vi "Preference_Panel.vi"(0 "Mode":T3) -> ()   [LabVIEW 2015]
uses:
  Anemometry Sub Vis/Controls/Server_Comms.ctl
  Anemometry Sub Vis/Controls/Preference_Mode.ctl
  Anemometry Sub Vis/Controls/EnFlo_Data_Folder_Setup.ctl
  Camera Server/Camera enum/Camera enum.ctl
  Anemometry Sub Vis/File/Setup_Filetype.ctl
  Anemometry Sub Vis/Controls/Overhead.ctl
  ADAM Client/Sub VIs/ADAM Controls/Ch_description_ADAM.ctl
  ADAM Client/Sub VIs/ADAM Controls/Module_type_ADAM.ctl
  ADAM Client/Sub VIs/ADAM Controls/Function_ADAM.ctl
  ADAM Client/Sub VIs/ADAM Controls/Channel_State.ctl
  ADAM Client/Sub VIs/ADAM Controls/Calib_type_ADAM.ctl
  ADAM Client/Sub VIs/ADAM Controls/Address.ctl
  Anemometry Sub Vis/Globals/Constants_global.vi
  Anemometry Sub Vis/Globals/Preference_global.vi
  Anemometry Sub Vis/Globals/Trav_pos_global.vi
  Camera Server/Globals/CamServer global.vi
  Anemometry Sub Vis/Acquisition/PWA/PWAtasksGLOBAL.vi
panel:
  in  "Cameras to Log":T1[](array[typedef])
  out "Preferences for computer":string
  in  "Log Cameras if available":bool
  in  "Use New Collision Code":bool
  in  "Traverse to Traverse Collision Detection":bool
  in  "DataTranslation Device No.":u32=20
  in  "Reset Email Counter":bool
  in  "EnFlo_Data_Folder_Setup":T2="EnFlo_Data on Server"
  in  "Post Processing Machine":bool
  in  "Analogue Device Serial No.":string="1188AB4"
  in  "PWA Device Serial No.":string="1187C98"
  in  "ADAM Setup File":u16(ring) items=["Current_Setup.xls"]
  in  "Default Source Establishment Time (s)":dbl=20.0
  out "This Machine's IP Number":string
  in  "Rig Setup":u16(ring) items=["3_x_2_tunnel", "A_Tunnel", "ADAM_Server", "Aero_Server", "Aero_Tunnel", "B_Tunnel", "Bench_Blower", "Contact_Conductance", "D_Tunnel", "EES_Project", "EnFlo_Tunnel", "Fruit_Rig", "Jet_Engine", "Laser_Disp_Scanner", "Paul_Hayden_Desk", "Post_Processing_Machine", "Soil_Rig", "Synthetic_Jet", "Tank", "TF_Standalone", "Wind_Turbine_Blade_Setup", "--New Rig Setup--"]
  in  "Default Traverse Name":u16(ring) items=["A_Tunnel", "Aero_Enclosure", "Aero_Sting", "Aero_ThroughWall", "Aero_Tunnel", "Angle_Calibrator", "B_Tunnel", "D_Tunnel", "dummy", "Dummy_Traverse", "EnFlo_", "EnFlo_Measure_Height", "EnFlo_Stack", "EnFlo_Stack  dfg", "EnFlo_Trav3", "EnFlo_Tunnel", "EnFlo_Turntable", "Fruit_Rig", "Hello_5.xls", "Laser_Disp_Scanner", "Laser_Meas_Traverse", "None", "Pitch_Traverse", "Pitch_Yaw", "PIV_Traverse", "Pressure_Port_1", "Pressure_Port_2", "Scanning Valve", "Soil_Rig", "Tank", "--New Traverse Setup--"]
  in  "OK":bool
  in  "% Error From First Calib":dbl=10.0 format="%.1f"
  in  "% Error From Previous Calib":dbl=0.5 format="%.1f"
  out "Templates":path=path "/G4_2_HD/Applications (Mac OS 9)/EnFlo Software/Anemometry/Anemometry Sub Vis/Templates"
  in  "Data Folder":path
  out "EnFlo SW Preferences":path=path "/G4_2_HD/Applications (Mac OS 9)/LabVIEW 5.1/EnFlo SW Preferences"
  in  "Tunnel Speed Control":bool
  in  "SMTP server IP address":string
  in  "Abs Press (mbar)":string="Froude:NPL:Atmos_Press"
  in  "Temperature":string="EnFlo Tun:Inlet Heater:Av Temp"
  in  "Server port number":u32=3363
  in  "Server address":string
  in  "LabVIEW Administrators":string[](array[string])=["", "", "", "", "", "", "", "", "", "", "", "", "", "", "", "", "", "", "", ""]
  in  "Server Comms":T4=enum."Do Not Link To Server"
  # "Server Computer Peferences"
  # "Multi Run Preferences"
  # "Warning Levels for Autocalibration Changes"
  # "Email Peferences"
  # "Deg C"
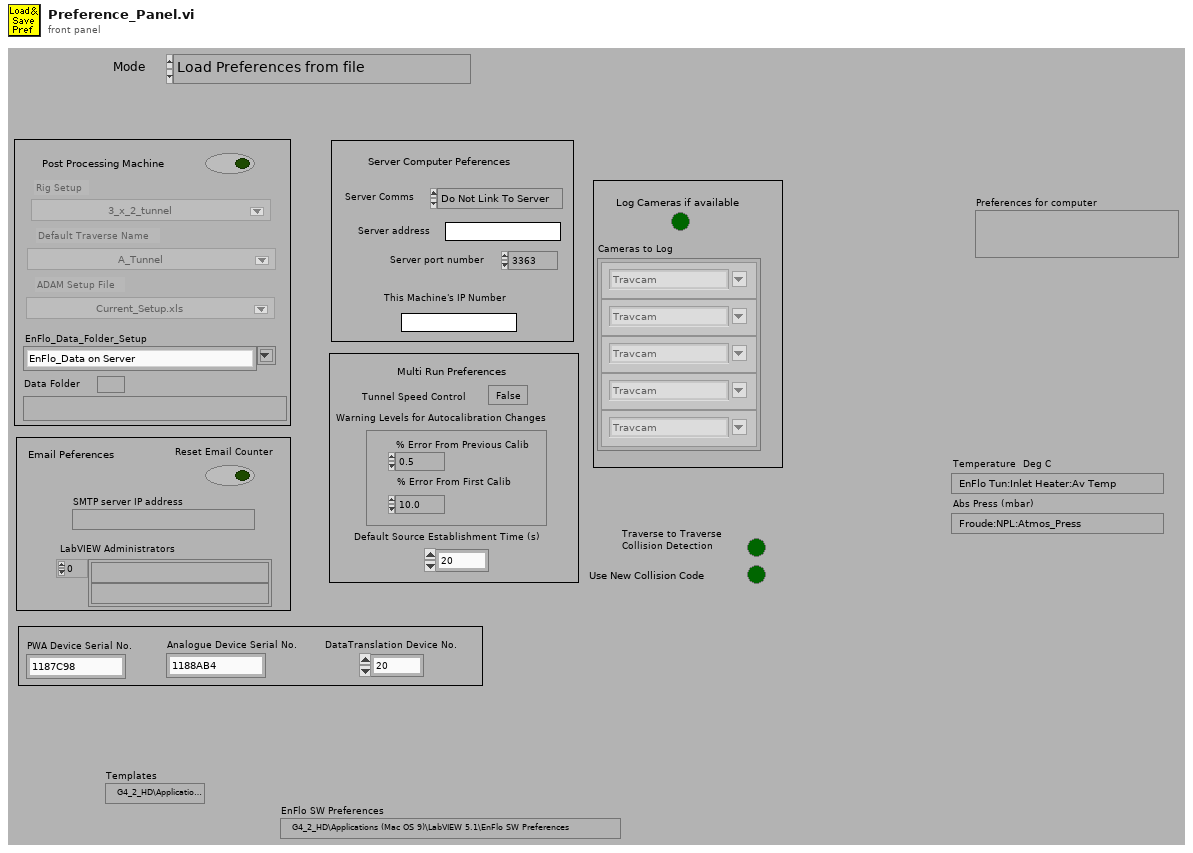
[diagram p1: front panel]
types:
  T1 = typedef "Camera enum.ctl" = string
  T2 = typedef "EnFlo_Data_Folder_Setup.ctl" = string
  T3 = typedef "Preference_Mode.ctl" = enum16{"Load Preferences from file", "Save Preferences to file", "Load, Edit then Save"}
  T4 = typedef "Server_Comms.ctl" = enum16{"Server Link Healthy", "Do Not Link To Server"}
  T5 = enum16{"Zero or one", "One", "Zero or more", "One or more"}
  T6 = enum8{"Enabled", "Disabled", "Disabled and Grayed Out"}
  T7 = typedef "Setup_Filetype.ctl" = enum16{"Measurement Setups", "Calibration Setups", "General", "Results File Plotter Setups", "Speed Calib Tweaks"}
  T8 = typedef "Overhead.ctl" = enum16{"Update total times", "Read Current Overhead", "Re Scale totals to 3 hrs", "Initialise totals to 3hr"}
  T9 = typedef "Calib_type_ADAM.ctl" = enum16{"Raw", "Bx + A", "Cx^2 + Bx + A", "Dx^3 + Cx^2 + Bx + A", "In Band", "Hi-Tec Q", "Hi-Tec M_dot", "Text"}
  T10 = typedef "Module_type_ADAM.ctl" = string
  T11 = typedef "Channel_State.ctl" = enum16{"On", "Off", "Always On", "Always Off"}
  T12 = typedef "LVDateTimeRec.ctl" = cluster{"fractional second":dbl, "second":i32, "minute":i32, "hour":i32, "day of month":i32, "month":i32, "year":i32, "day of week":i32, "day of year":i32, "DST":i32}
  T13 = typedef "Ch_description_ADAM.ctl" = cluster{"Ch Name":string, "Type":T10, "Function":T14, "Ch State":T11, "Calibration type":T9, "A":dbl, "B":dbl, "C":dbl, "D":dbl, "Comments":string, "Address":T15, "String":string, "Duty":u16}
  T14 = typedef "Function_ADAM.ctl" = enum16{"Analogue Input", "Digital Input", "Event counter", "Event rate", "Analogue Output", "Digital Output", "Relay Output"}
  T15 = typedef "Address.ctl" = cluster{"Main":i32, "Ch.":i32, "Sub":i32, "Port Name":string}
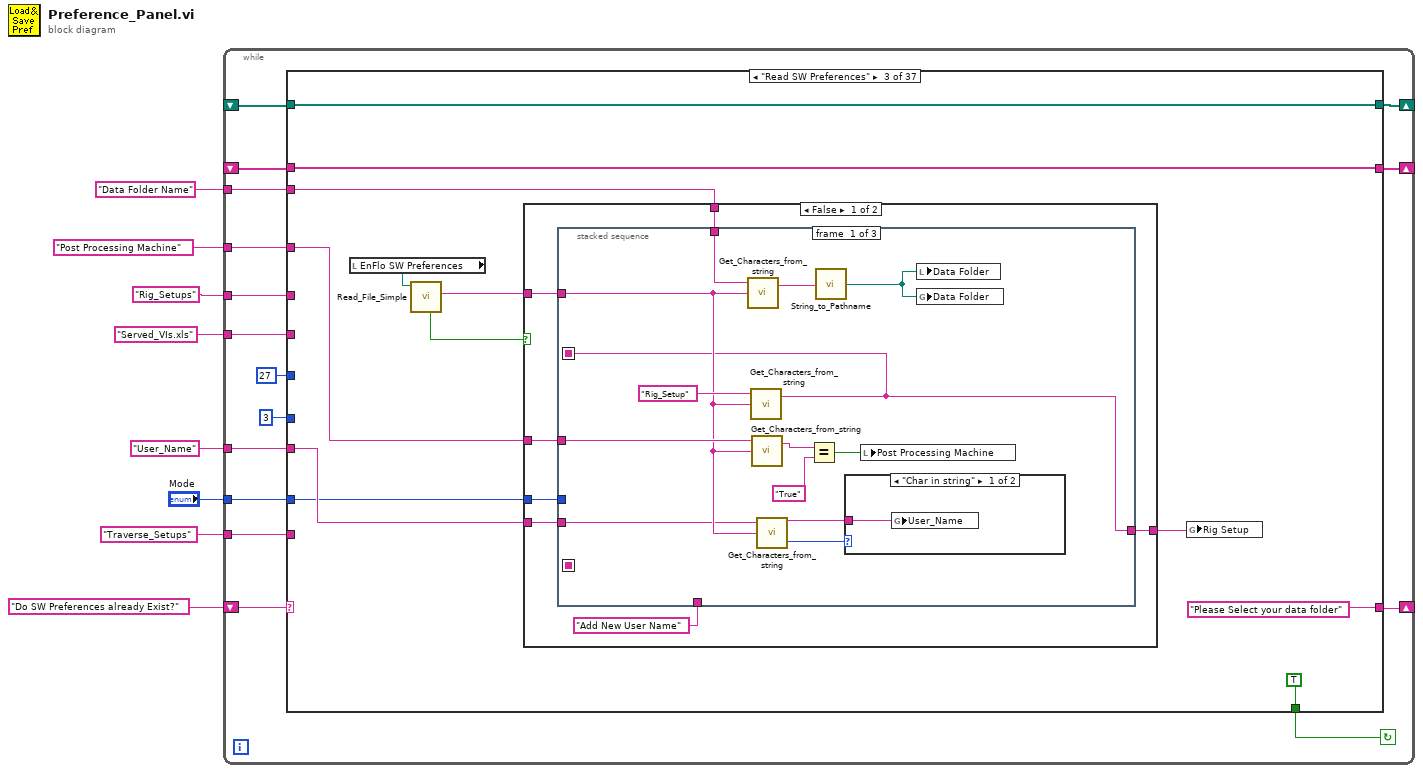
[diagram p0: block diagram]
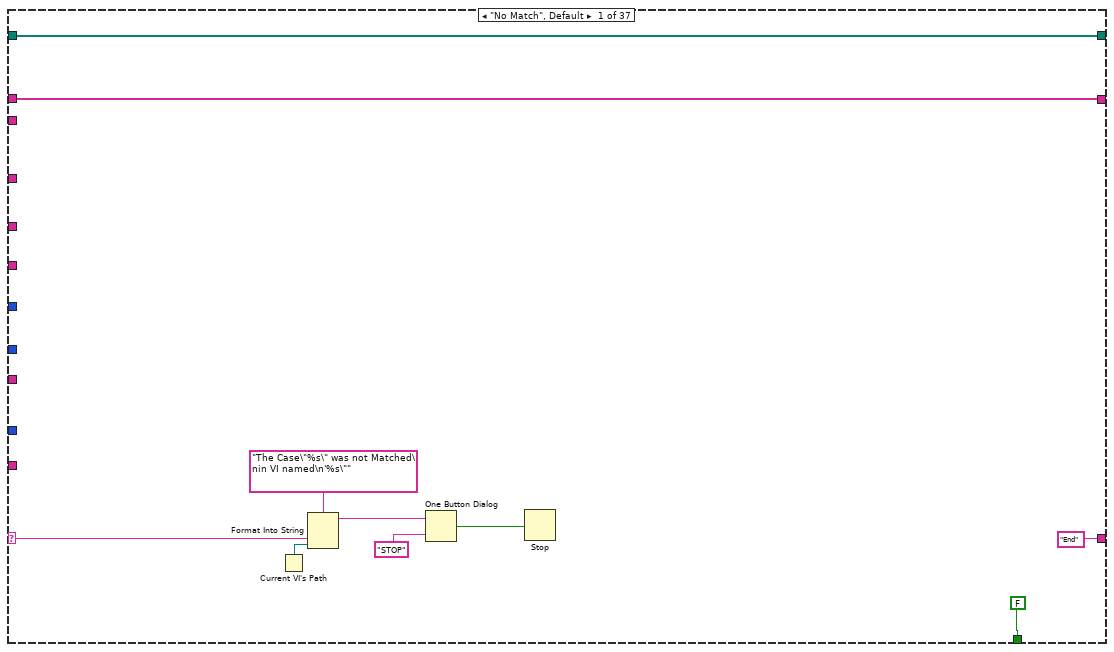
[diagram p2: hidden frame]
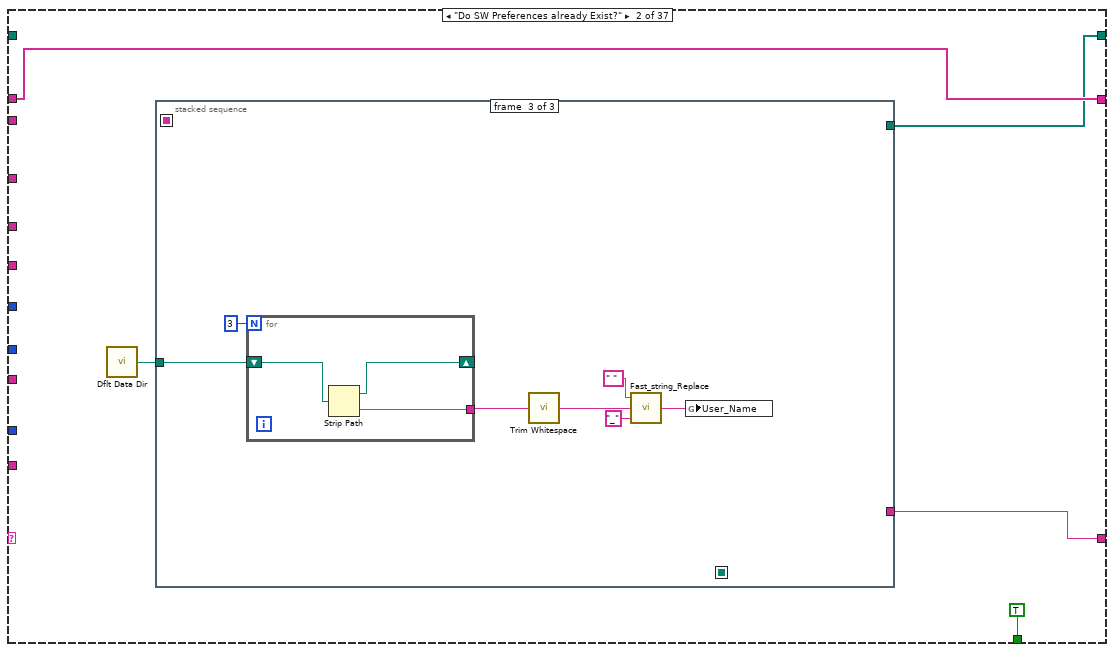
[diagram p3: hidden frame]
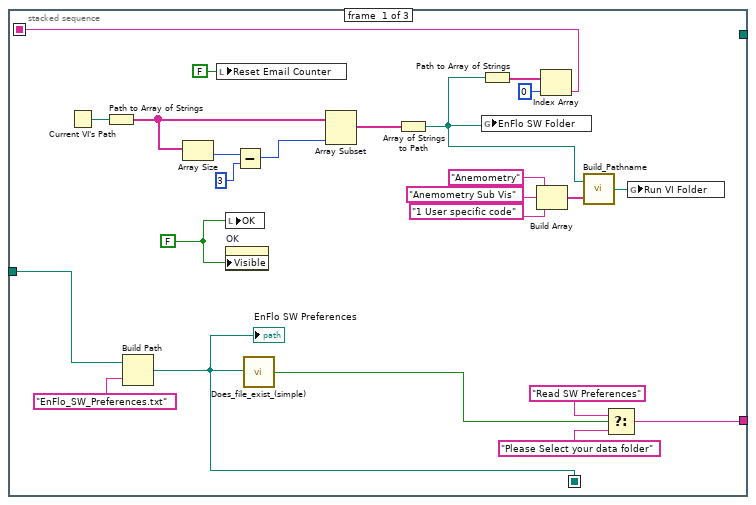
[diagram p4: hidden frame]
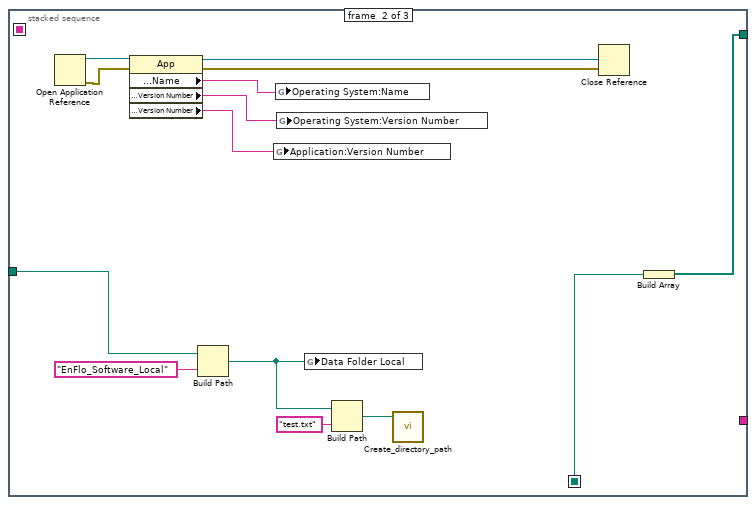
[diagram p5: hidden frame]
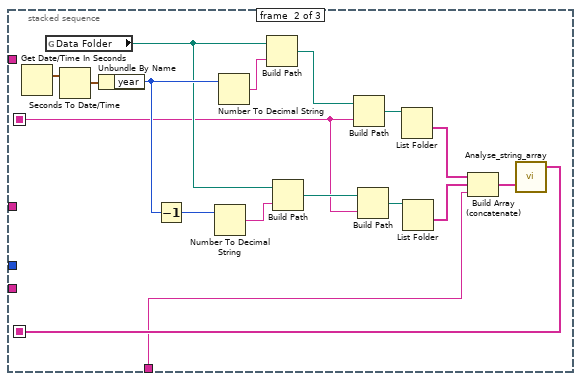
[diagram p7: hidden frame]
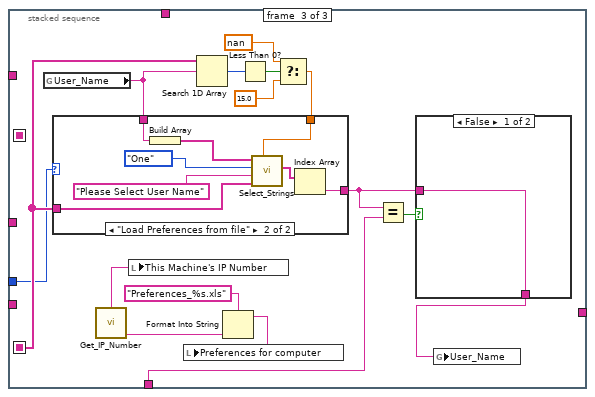
[diagram p8: hidden frame]
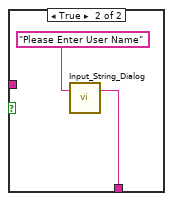
[diagram p10: hidden frame]
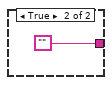
[diagram p11: hidden frame]
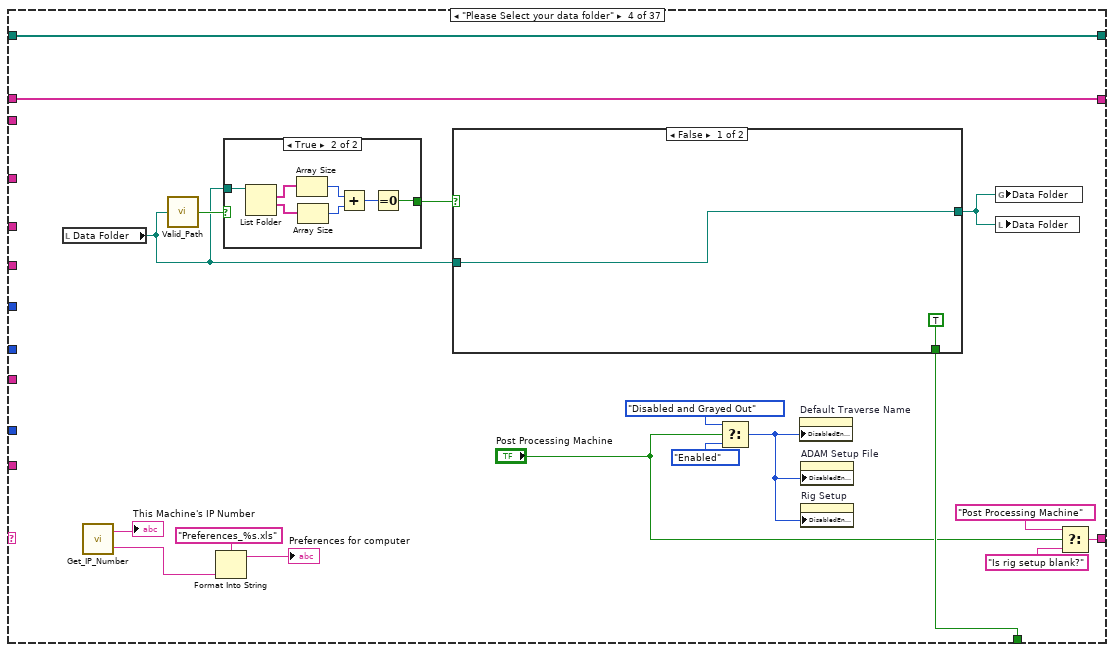
[diagram p12: hidden frame]
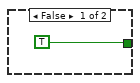
[diagram p13: hidden frame]
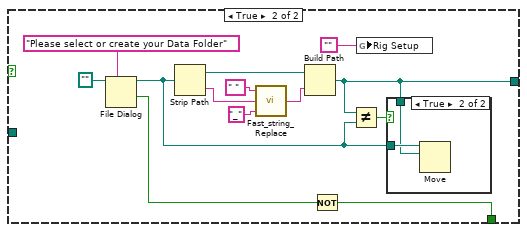
[diagram p14: hidden frame]
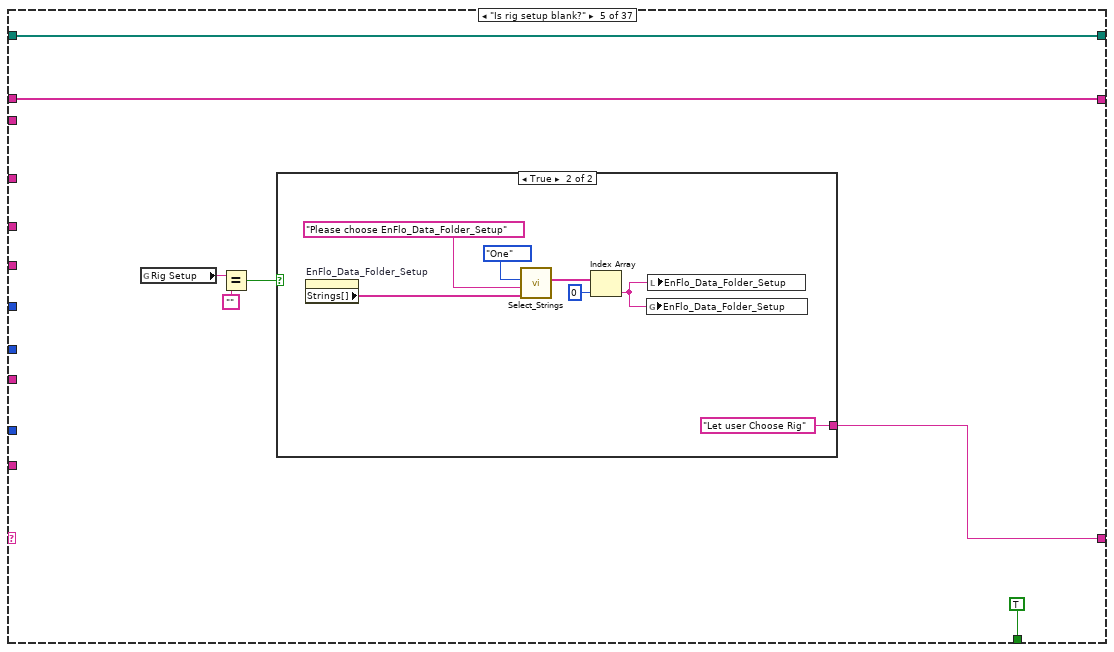
[diagram p16: hidden frame]
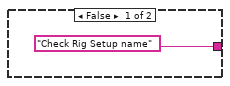
[diagram p17: hidden frame]
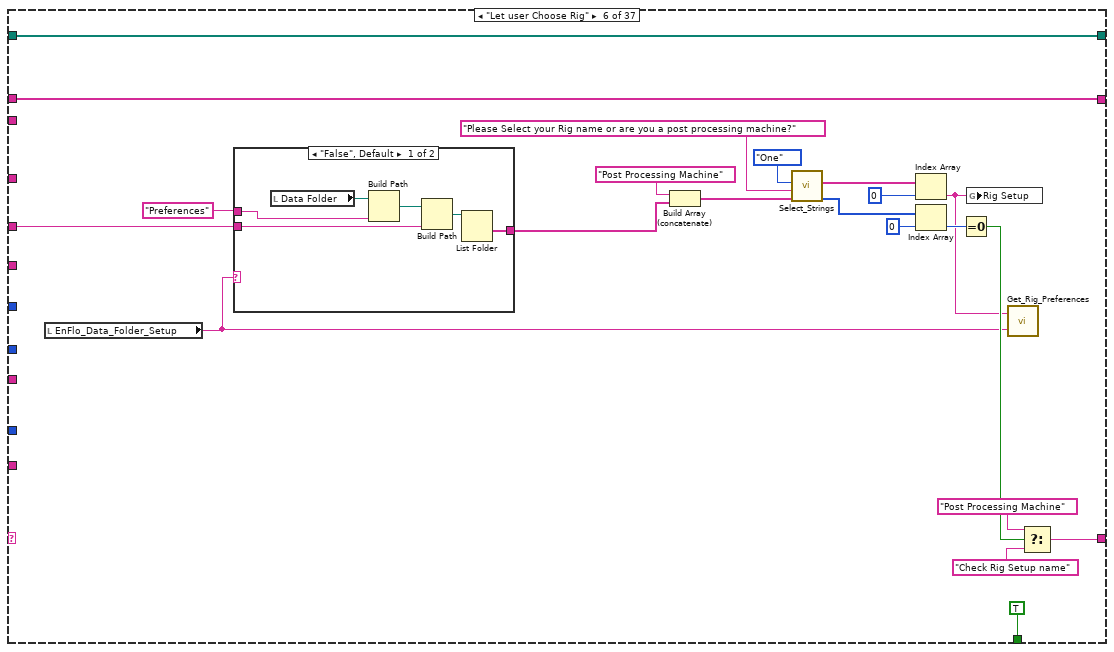
[diagram p18: hidden frame]
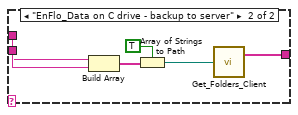
[diagram p19: hidden frame]
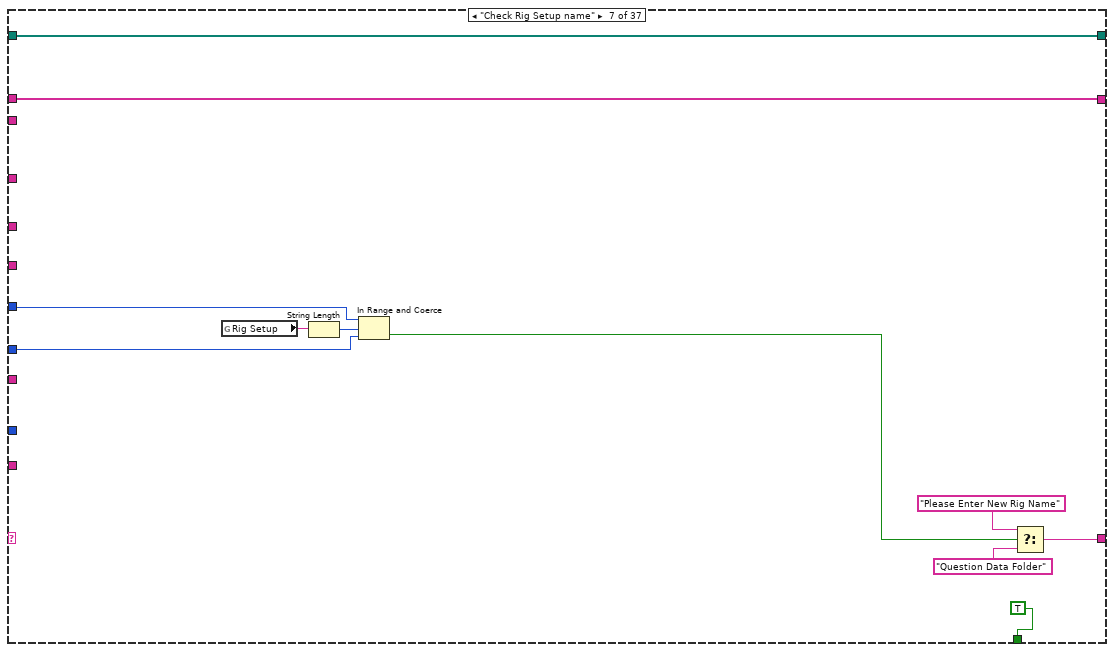
[diagram p20: hidden frame]
diagram:
  n1 = while {
    shift-left: _ -> [w21]
    shift-right: [w22] -> _
    shift-left: "Do SW Preferences already Exist?" -> [w10]
    shift-right: [w23] -> _
    tunnel: "Mode" -> [w20]
    tunnel: "Data Folder Name" ("Label for characters") -> [w19]
    tunnel: "Served_VIs.xls" ("Substring") -> [w18]
    tunnel: "Rig_Setups" ("Folder") -> [w15]
    tunnel: "Traverse_Setups" ("name or relative path") -> [w14]
    shift-right: [w13] -> _
    shift-left: _ -> [w12]
    tunnel: "Post Processing Machine" ("Label for characters") -> [w11]
    tunnel: "User_Name" ("Label for characters") -> [w9]
    stop <- w24 continue-if-true
    n2 = case shown="\"Read SW Preferences\"" w10 {
      selector: w10 -> [w25 _ _ _ _ _ _ _ _ _ _ _ _ _ _ _ _ _ _ _ _ _ _ _ _ _ _ _ _ _ _ _ _ _ _ _ _]
      tunnel: [FALSE TRUE TRUE w178 TRUE TRUE TRUE TRUE TRUE TRUE TRUE TRUE TRUE TRUE TRUE TRUE TRUE TRUE TRUE TRUE TRUE TRUE TRUE TRUE TRUE TRUE TRUE TRUE TRUE TRUE TRUE TRUE w940 TRUE TRUE TRUE FALSE] -> w24
      tunnel: ["End" w37 "Please Select your data folder" w175 w210 w241 w258 w269 w288 "Update Constants Global" ("f") "Copy Preferences?" "Copy Preferences?" w419 w436 "Install Preference files" "Install Adam table files" "Install Adam setup files" "Choose ADAM Setup file" "Preference files continued" "Variable Names" w613 w633 "Please Enter new  Traverse Setup" w720 "Create Traverse setup" ("f") "Check file permission status" w817 w848 w868 w888 w904 "Save Preference File" "Save SW Preferences" w1030 w1044 "Initialise Globals" "End"] -> w23
      tunnel: [w27 w38 w98 w184 w215 w244 w267 w277 w290 w355 w383 w406 w417 w439 w495 w510 w535 w554 w576 w586 w618 w640 w708 w722 w756 w773 w818 w853 w873 w896 w909 w929 w946 w1038 w1045 w1097 w1155] -> w22
      tunnel: w21 -> [w27 w38 w98 w184 w215 w244 w267 w277 w290 w355 w383 w406 w417 w439 w495 w510 w535 w554 w576 w586 _ w640 w708 w722 w756 w773 w818 w853 w873 w896 w909 w929 w946 w1038 w1045 w1097 w1155]
      tunnel: w20 -> [_ _ w88 _ _ _ _ _ _ _ _ _ _ _ _ _ _ _ _ _ w612 _ _ _ _ _ w816 _ _ _ _ _ w941 _ _ _ _]
      tunnel: w19 -> [_ _ w95 _ _ _ _ _ _ _ _ _ _ _ _ _ _ _ _ _ _ _ _ _ _ _ _ _ _ _ _ _ _ w1029 _ _ _]
      tunnel: w18 -> [_ _ _ _ _ _ _ _ _ _ _ _ _ _ _ w505 _ _ _ _ _ _ _ _ _ _ _ _ _ _ _ _ _ _ _ w1089 _]
      tunnel: 3 ("lower limit") -> [_ _ _ _ _ _ w263 _ w287 _ _ _ _ _ _ _ _ _ _ _ _ _ _ w719 _ _ _ _ _ _ _ _ _ _ _ _ _]
      tunnel: 27 ("upper limit") -> [_ _ _ _ _ _ w264 _ w286 _ _ _ _ _ _ _ _ _ _ _ _ _ _ w718 _ _ _ _ _ _ _ _ _ _ _ _ _]
      tunnel: w15 -> [_ _ _ _ _ w229 _ _ _ w343 w372 _ _ _ _ _ _ _ _ _ _ _ _ _ _ _ _ _ _ _ _ _ _ _ _ _ _]
      tunnel: w14 -> [_ _ _ _ _ _ _ _ _ _ _ _ _ _ _ _ _ _ _ _ _ _ w706 _ w743 _ _ _ _ _ _ _ _ _ _ _ _]
      tunnel: [w26 w35 w94 w179 w211 w243 w266 w276 w282 w341 w369 w396 w418 w440 w488 w502 w528 w551 w562 w578 w605 w636 w705 w714 w742 w769 path[] [] w845 w865 w891 w907 w928 w939 w1026 w1043 w1091 w1153] -> w13
      tunnel: w12 -> [w26 _ w94 w179 w211 w243 w266 w276 w282 w341 w369 w396 w418 w440 w487 w504 w528 w552 w562 w580 w605 w637 w705 w714 w742 w770 w815 w845 w865 w891 w907 w928 w939 w1026 w1043 w1091 w1153]
      tunnel: w11 -> [_ _ w93 _ _ _ _ _ _ _ _ _ _ _ _ _ _ _ _ _ _ _ _ _ _ _ _ _ _ _ _ _ _ w1020 _ _ _]
      tunnel: w9 -> [_ _ w89 _ _ _ _ _ _ _ _ _ _ _ _ _ _ _ _ _ _ _ _ _ _ _ _ _ _ _ _ _ _ w1019 _ _ _]
      frame "No Match", Default {
        n3 = Current VI's Path() -> (path=w34:path)
        n4 = Format Into String(format string="The Case\"%s\" was not Matched\nin VI named\n'%s\"" ("Format String"), w25, w34) -> (resulting string=w31:string)  [unwired: 2 in, 1 out]
        n5 = One Button Dialog(message=w31, button name ("OK")="STOP") -> (true=w33:bool)
        n6 = Stop(stop? (T)=w33) -> ()
      }
      frame "Do SW Preferences already Exist?" {
        n7 = call <vilib>:"Dflt Data Dir.vi"() -> ("App:Default Data Directory"=w36:path)
        n8 = stacked-sequence {
          seq-local: [w50 _ _] -> [_ _ _]
          seq-local: [w48 _ _] -> [_ w69 _]
          tunnel: [w53 _ _] -> w37
          tunnel: w36 -> [w49 w67 w83]
          tunnel: [_ w70 _] -> w35
          frame #0 {
            w47 = FALSE ("OK")
            n9 = Current VI's Path() -> (path=w61:path)
            n10 = Path to Array of Strings(0:w61) -> (2:w58:string[])  [unwired: 1 out]
            n11 = Build Path(base path=w49, name or relative path="EnFlo_SW_Preferences.txt") -> (appended path=w48:path)
            "EnFlo SW Preferences" <- w48
            n12 = Array Size(array=w58) -> (size(s)=w60:i32)
            n13 = local write "Reset Email Counter"(FALSE ("Reset Email Counter")) -> ()
            n14 = local write "OK"(w47) -> ()
            n15 = property on="OK" class="Bool (strict)"("Visible"=w47) -> ()  [unwired: 2 in, 2 out]
            n16 = Subtract(x=w60, y=3) -> (x-y=w56:i32)
            n17 = call "Does_file_exist_(simple).vi"("Pathname"=w48) -> ("exists?"=w62:bool)
            n18 = Array Subset(array=w58, length=w56) -> (w57:string[])  [unwired: 1 in]
            n19 = Array of Strings to Path(0:w57) -> (2:w45:path)  [unwired: 1 out]
            n20 = Path to Array of Strings(0:w45) -> (2:w51:string[])  [unwired: 1 out]
            n21 = global write "Constants_global.vi" "EnFlo SW Folder"(w45) -> ()
            n22 = Build Array("Anemometry" ("name or relative path"), "Anemometry Sub Vis" ("name or relative path"), "1 User specific code" ("name or relative path")) -> (w40:string[])
            n23 = Index Array(array=w51, index=0) -> (element=w50:string)
            n24 = call "Build_Pathname.vi"("PathElements"=w40, "PathnameIn"=w45) -> ("AppendedPath"=w44:path)
            n25 = Select(t="Read SW Preferences", s=w62, f="Please Select your data folder") -> (s? t:f=w53:string)
            n26 = global write "Constants_global.vi" "Run VI Folder"(w44) -> ()
          }
          frame #1 {
            n27 = Open Application Reference() -> (0:w74:errorcluster, 3:w77:refnum<vi>)  [unwired: 1 in, 3 out]
            n28 = property class="App"(reference=w77, error in=w74) -> (reference out=w76:refnum<vi>, error out=w75:errorcluster, "Operating System:Name"=w71:string, "Operating System:Version Number"=w73:string, "Application:Version Number"=w72:string)
            n29 = Build Path(base path=w67, name or relative path="EnFlo_Software_Local" ("element")) -> (appended path=w66:path)
            n30 = global write "Preference_global.vi" "Application:Version Number"(w72) -> ()
            n31 = global write "Preference_global.vi" "Operating System:Name"(w71) -> ()
            n32 = global write "Preference_global.vi" "Operating System:Version Number"(w73) -> ()
            n33 = global write "Constants_global.vi" "Data Folder Local"(w66) -> ()
            n34 = Build Path(base path=w66, name or relative path="test.txt") -> (appended path=w64:path)
            n35 = call "Create_directory_path.vi"("Path name"=w64) -> ()  [unwired: 2 in, 2 out]
            n36 = Close Reference(reference=w76, error in (no error)=w75) -> ()  [unwired: 1 out]
            n37 = Build Array(w69) -> (w70:path[])
          }
          frame #2 {
            n38 = for {
              N: 3 -> [_]
              shift-right: [w87] -> _
              shift-left: w83 -> [w86]
              tunnel: [w85] -> w79
              n39 = Strip Path(path=w86) -> (stripped path=w87:path, name=w85:string)
            }
            n40 = call <vilib>:"Trim Whitespace.vi"("string"=w79) -> ("trimmed string"=w78:string)  [unwired: 1 in]
            n41 = call "Fast_string_Replace.vi"("Replace match with:"="_", "Input String"=w78, "regular expression"=" ") -> ("Output String"=w80:string)  [unwired: 1 in, 1 out]
            n42 = global write "Preference_global.vi" "User_Name"(w80) -> ()
          }
        }
      }
      frame "Read SW Preferences" {
        n43 = local read "EnFlo SW Preferences"() -> (w97:path)
        n44 = call "Read_File_Simple.vi"("Filename"=w97) -> ("Error?"=w91:bool, "string"=w92:string)  [unwired: 2 in, 6 out]
        n45 = case shown="False" w91 {
          tunnel: w95 -> [w106 _]
          tunnel: w93 -> [w105 _]
          tunnel: w92 -> [w103 _]
          tunnel: [w104 ""] -> w90
          tunnel: w89 -> [w102 _]
          tunnel: w88 -> [w100 _]
          frame False {
            n46 = stacked-sequence {
              seq-local: [w109 _ _] -> [_ w127 _]
              seq-local: [_ w122 _] -> [_ _ w148]
              tunnel: w106 -> [w119 _ _]
              tunnel: w105 -> [w117 _ _]
              tunnel: [w109 _ _] -> w104
              tunnel: w103 -> [w113 _ _]
              tunnel: w102 -> [w112 _ _]
              tunnel: "Add New User Name" -> [_ w121 w153]
              tunnel: w100 -> [_ _ w138]
              frame #0 {
                n47 = call "Get_Characters_from_string.vi"("Input string"=w113, "Variable name"=w119) -> ("Value"=w108:string)  [unwired: 1 in, 1 out]
                n48 = call "Get_Characters_from_string.vi"("Input string"=w113, "Variable name"="Rig_Setup" ("Label for characters")) -> ("Value"=w109:string)  [unwired: 1 in, 1 out]
                n49 = call "Get_Characters_from_string.vi"("Input string"=w113, "Variable name"=w117) -> ("Value"=w116:string)  [unwired: 1 in, 1 out]
                n50 = call "Get_Characters_from_string.vi"("Input string"=w113, "Variable name"=w112) -> ("Status"=w111:enum16{"Char in string", "Char not in string"}, "Value"=w110:string)  [unwired: 1 in]
                n51 = Equal?(x=w116, y="True") -> (x = y?=w114:bool)
                n52 = call "String_to_Pathname.vi"("Input String"=w108) -> ("path"=w107:path)
                n53 = case shown="\"Char in string\"" w111 {
                  tunnel: w110 -> [w120 _]
                  frame "Char in string" {
                    n54 = global write "Preference_global.vi" "User_Name"(w120) -> ()
                  }
                  frame "Char not in string" {
                  }
                }
                n55 = local write "Post Processing Machine"(w114) -> ()
                n56 = local write "Data Folder"(w107) -> ()
                n57 = global write "Constants_global.vi" "Data Folder"(w107) -> ()
              }
              frame #1 {
                n58 = Get Date/Time In Seconds() -> (seconds since 1Jan1904=w137:timestamp)
                n59 = global read "Constants_global.vi" "Data Folder"() -> (w130:path)
                n60 = Seconds To Date/Time(time stamp (now)=w137) -> (date time rec=w136:T12)  [unwired: 1 in]
                n61 = Unbundle By Name(w136) -> ("year"=w135:i32)
                n62 = Decrement(x=w135) -> (x-1=w134:i32)
                n63 = Number To Decimal String(number=w134) -> (decimal integer string=w129:string)  [unwired: 1 in]
                n64 = Number To Decimal String(number=w135) -> (decimal integer string=w133:string)  [unwired: 1 in]
                n65 = Build Path(base path=w130, name or relative path=w133) -> (appended path=w132:path)
                n66 = Build Path(base path=w130, name or relative path=w129) -> (appended path=w128:path)
                n67 = Build Path(base path=w132, name or relative path=w127) -> (appended path=w131:path)
                n68 = Build Path(base path=w128, name or relative path=w127) -> (appended path=w126:path)
                n69 = List Folder(path=w131) -> (folder names=w125:string[])  [unwired: 3 in, 3 out]
                n70 = List Folder(path=w126) -> (folder names=w124:string[])  [unwired: 3 in, 3 out]
                n71 = Build Array (concatenate)(w125, w124, w121) -> (w123:string[])
                n72 = call "Analyse_string_array.vi"("String array"=w123) -> ("Unique strings"=w122:string[])  [unwired: 1 in, 1 out]
              }
              frame #2 {
                n73 = global read "Preference_global.vi" "User_Name"() -> (w149:string)
                n74 = call "Get_IP_Number.vi"() -> ("Computer Name"=w141:string, "IP Number"=w142:string)
                n75 = local write "This Machine's IP Number"(w142) -> ()
                n76 = Search 1D Array(1D array=w148, element=w149) -> (index of element=w147:i32)  [unwired: 1 in]
                n77 = Format Into String(format string="Preferences_%s.xls" ("name or relative path"), w141) -> (resulting string=w140:string)  [unwired: 2 in, 1 out]
                n78 = local write "Preferences for computer"(w140) -> ()
                n79 = Less Than 0?(x=w147) -> (x < 0?=w146:bool)
                n80 = Select(t=nan ("Timeout (s)"), s=w146, f=15.0 ("Timeout (s)")) -> (s? t:f=w143:dbl)
                n81 = case shown="\"Load Preferences from file\"" w138 {
                  tunnel: [w154 w158] -> w150
                  tunnel: w149 -> [w154 w157]
                  tunnel: w148 -> [_ w156]
                  tunnel: w143 -> [_ w155]
                  frame Default {
                  }
                  frame "Load Preferences from file" {
                    n82 = Build Array(w157) -> (w161:string[])
                    n83 = call "Select_Strings.vi"("Timeout (s)"=w155, "Available Ch names"=w156, "Message"="Please Select User Name", "Selector mode"=T5."One", "Desired Ch names (in)"=w161) -> ("Selected Channel Names"=w159:string[])  [unwired: 1 in, 2 out]
                    n84 = Index Array(array=w159) -> (element=w158:string)  [unwired: 1 in]
                  }
                }
                n85 = Equal?(x=w150, y=w153) -> (x = y?=w152:bool)
                n86 = case shown="False" w152 {
                  tunnel: [w163 w164] -> w151
                  tunnel: w150 -> [w163 _]
                  frame False {
                  }
                  frame True {
                    n87 = call "Input_String_Dialog.vi"("Message to user"="Please Enter User Name") -> ("Output string"=w164:string)  [unwired: 1 in, 1 out]
                  }
                }
                n88 = global write "Preference_global.vi" "User_Name"(w151) -> ()
              }
            }
          }
          frame True {
          }
        }
        n89 = global write "Preference_global.vi" "Rig Setup"(w90) -> ()
      }
      frame "Please Select your data folder" {
        n90 = local read "Data Folder"() -> (w180:path)
        n91 = call "Get_IP_Number.vi"() -> ("Computer Name"=w169:string, "IP Number"=→"This Machine's IP Number":string)
        n92 = call "Valid_Path.vi"("Filename"=w180) -> ("Valid Path?"=w182:bool)
        n93 = Format Into String(format string="Preferences_%s.xls" ("name or relative path"), w169) -> (resulting string=→"Preferences for computer":string)  [unwired: 2 in, 1 out]
        n94 = case shown="True" w182 {
          tunnel: [TRUE ("status") w186] -> w181
          tunnel: w180 -> [_ w192]
          frame False {
          }
          frame True {
            n95 = List Folder(path=w192) -> (filenames=w190:string[], folder names=w191:string[])  [unwired: 1 in, 4 out]
            n96 = Array Size(array=w190) -> (size(s)=w188:i32)
            n97 = Array Size(array=w191) -> (size(s)=w189:i32)
            n98 = Add(x=w188, y=w189) -> (x+y=w187:i32)
            n99 = Equal To 0?(x=w187) -> (x = 0?=w186:bool)
          }
        }
        n100 = case shown="False" w181 {
          tunnel: [w194 w198] -> w183
          tunnel: w180 -> [w194 _]
          tunnel: [TRUE w196] -> w178
          frame False {
          }
          frame True {
            n101 = File Dialog(7:"Please select or create your Data Folder" ("prompt"), 11:path "") -> (1:w197:bool, 3:w199:path)  [unwired: 1 in, 6 out]
            n102 = Strip Path(path=w199) -> (stripped path=w203:path, name=w202:string)
            n103 = call "Fast_string_Replace.vi"("Replace match with:"="_", "Input String"=w202, "regular expression"=" ") -> ("Output String"=w201:string)  [unwired: 2 out]
            n104 = Build Path(base path=w203, name or relative path=w201) -> (appended path=w198:path)
            n105 = Not(x=w197) -> (.not. x?=w196:bool)
            n106 = Not Equal?(x=w198, y=w199) -> (x != y?=w200:bool)
            n107 = global write "Preference_global.vi" "Rig Setup"("") -> ()
            n108 = case shown="True" w200 {
              tunnel: w199 -> [_ w209]
              tunnel: w198 -> [_ w208]
              frame False {
              }
              frame True {
                n109 = Move(source path=w209, 10:w208) -> ()  [unwired: 1 in, 5 out]
              }
            }
          }
        }
        n110 = Select(t=T6."Disabled and Grayed Out" ("Disabled"), s="Post Processing Machine", f=T6."Enabled" ("Disabled")) -> (s? t:f=w171:T6)
        n111 = property on="Default Traverse Name" class="Ring (strict)"("DisabledEnum"=w171) -> ()  [unwired: 2 in, 2 out]
        n112 = property on="ADAM Setup File" class="Ring (strict)"("DisabledEnum"=w171) -> ()  [unwired: 2 in, 2 out]
        n113 = property on="Rig Setup" class="Ring (strict)"("DisabledEnum"=w171) -> ()  [unwired: 2 in, 2 out]
        n114 = global write "Constants_global.vi" "Data Folder"(w183) -> ()
        n115 = local write "Data Folder"(w183) -> ()
        n116 = Select(t="Post Processing Machine", s="Post Processing Machine", f="Is rig setup blank?") -> (s? t:f=w175:string)
      }
      frame "Is rig setup blank?" {
        n117 = global read "Preference_global.vi" "Rig Setup"() -> (w212:string)
        n118 = Equal?(x=w212, y="") -> (x = y?=w213:bool)
        n119 = case shown="True" w213 {
          tunnel: ["Check Rig Setup name" ("t") "Let user Choose Rig"] -> w210
          frame False {
          }
          frame True {
            n120 = property on="EnFlo_Data_Folder_Setup" class="CmbBox (strict)"() -> ("Strings[]"=w222:string[])  [unwired: 2 in, 2 out]
            n121 = call "Select_Strings.vi"("Available Ch names"=w222, "Message"="Please choose EnFlo_Data_Folder_Setup", "Selector mode"=T5."One") -> ("Selected Channel Names"=w220:string[])  [unwired: 3 in, 2 out]
            n122 = Index Array(array=w220, index=0) -> (element=w218:string)
            n123 = global write "Preference_global.vi" "EnFlo_Data_Folder_Setup"(w218) -> ()
            n124 = local write "EnFlo_Data_Folder_Setup"(w218) -> ()
          }
        }
      }
      frame "Let user Choose Rig" {
        n125 = local read "EnFlo_Data_Folder_Setup"() -> (w225:T2)
        n126 = case shown="\"False\", Default" w225 {
          tunnel: "Preferences" ("name or relative path") -> [w249 w252]
          tunnel: w229 -> [w248 w257]
          tunnel: [w247 w254] -> w227
          frame "False", Default {
            n127 = local read "Data Folder"() -> (w250:path)
            n128 = Build Path(base path=w250, name or relative path=w249) -> (appended path=w251:path)
            n129 = Build Path(base path=w251, name or relative path=w248) -> (appended path=w246:path)
            n130 = List Folder(path=w246) -> (folder names=w247:string[])  [unwired: 1 in, 5 out]
          }
          frame "EnFlo_Data on C drive - backup to server" {
            n131 = Build Array(w252, w257) -> (w256:string[])
            n132 = Array of Strings to Path(0:w256, 1:TRUE ("relative")) -> (2:w253:path)
            n133 = call "Get_Folders_Client.vi"("Relative Path"=w253) -> ("Folder Names"=w254:string[])  [unwired: 1 out]
          }
        }
        n134 = Build Array (concatenate)("Post Processing Machine", w227) -> (w234:string[])
        n135 = call "Select_Strings.vi"("Available Ch names"=w234, "Message"="Please Select your Rig name or are you a post processing machine?", "Selector mode"=T5."One") -> ("Ch Indicies Choosen"=w231:i32[], "Selected Channel Names"=w233:string[])  [unwired: 3 in, 1 out]
        n136 = Index Array(array=w233, index=0) -> (element=w226:string)
        n137 = Index Array(array=w231, index=0) -> (element=w230:i32)
        n138 = Equal To 0?(x=w230) -> (x = 0?=w240:bool)
        n139 = global write "Preference_global.vi" "Rig Setup"(w226) -> ()
        n140 = call "Get_Rig_Preferences.vi"("EnFlo_Data_Folder_Setup"=w225, "Rig Setup"=w226) -> ()  [unwired: 1 in]
        n141 = Select(t="Post Processing Machine", s=w240, f="Check Rig Setup name") -> (s? t:f=w241:string)
      }
      frame "Check Rig Setup name" {
        n142 = global read "Preference_global.vi" "Rig Setup"() -> (w259:string)
        n143 = String Length(string=w259) -> (length=w265:i32)
        n144 = In Range and Coerce(upper limit=w264, x=w265, lower limit=w263) -> (In Range?=w262:bool)  [unwired: 1 out]
        n145 = Select(t="Please Enter New Rig Name", s=w262, f="Question Data Folder") -> (s? t:f=w258:string)
      }
      frame "Question Data Folder" {
        n146 = local read "Data Folder"() -> (w275:path)
        n147 = Format Into String(format string="Is the Data Folder\n%s\nCorrect?" ("message"), w275) -> (resulting string=w273:string)  [unwired: 2 in, 1 out]
        n148 = Two Button Dialog(message=w273, 1:"No, let me change it" ("F button name (\"Cancel\")"), 2:"Yes" ("T button name (\"OK\")")) -> (T button?=w270:bool)
        n149 = case shown="True" w270 {
          tunnel: ["Please Select your data folder" "Please Enter New Rig Name"] -> w269
          frame False {
            n150 = local write "Data Folder"(path "") -> ()
          }
          frame True {
          }
        }
      }
      frame "Please Enter New Rig Name" {
        n151 = global read "Preference_global.vi" "Rig Setup"() -> (w284:string)
        n152 = String Length(string=w284) -> (length=w289:i32)
        n153 = In Range and Coerce(upper limit=w286, x=w289, lower limit=w287) -> (In Range?=w285:bool)  [unwired: 1 out]
        n154 = case shown="False" w285 {
          tunnel: w284 -> [w296 w339]
          tunnel: [w292 "Update Rig setup menu ring"] -> w288
          tunnel: [w293 w339] -> w283
          tunnel: w287 -> [w295 _]
          tunnel: w286 -> [w294 _]
          frame False {
            n155 = stacked-sequence {
              seq-local: [w297 _] -> [_ w322]
              seq-local: [w304 _] -> [_ _]
              tunnel: w296 -> [w306 _]
              tunnel: w295 -> [w317 _]
              tunnel: w294 -> [w303 w320]
              tunnel: [_ w325] -> w293
              tunnel: [w309 _] -> w292
              frame #0 {
                n156 = Match Pattern(string=w306, regular expression="-") -> (before substring=w305:string, after substring=w304:string)  [unwired: 3 out]
                n157 = String Length(string=w304) -> (length=w302:i32)
                n158 = Subtract(x=w303, y=w302) -> (x-y=w301:i32)
                n159 = Format Into String(format string="Please Enter a Rig Name.\n It must be between %d and %d Characters" ("Message to user"), w317, w301) -> (resulting string=w316:string)  [unwired: 2 in, 1 out]
                n160 = call "Input_String_Dialog.vi"("Value"=w305, "Message to user"=w316) -> ("Ok Out"=w312:bool, "Output string"=w313:string)
                n161 = call "Fast_string_Replace.vi"("Replace match with:"="_", "Input String"=w313, "regular expression"=" ") -> ("Output String"=w298:string)  [unwired: 2 out]
                n162 = Select(t="Please Enter New Rig Name", s=w312, f="Save Preference File") -> (s? t:f=w309:string)
                n163 = call "Fast_string_Replace.vi"("Replace match with:"="_", "Input String"=w298, "regular expression"="-") -> ("Output String"=w297:string)  [unwired: 2 out]
              }
              frame #1 {
                n164 = String Length(string=w322) -> (length=w321:i32)
                n165 = Subtract(x=w320, y=w321) -> (x-y=w319:i32)
                n166 = Format Into String(format string="Please Enter a Rig Machine identifier if more than one machine per Rig.\n(Leave Blank for Rigs only using one Machine.)\nMust be less than %d Characters." ("Message to user"), w319) -> (resulting string=w318:string)  [unwired: 2 in, 1 out]
                n167 = call "Input_String_Dialog.vi"("Value"="", "Message to user"=w318) -> ("Output string"=w331:string)  [unwired: 1 out]
                n168 = call "Fast_string_Replace.vi"("Replace match with:"="_", "Input String"=w331, "regular expression"=" ") -> ("Output String"=w327:string)  [unwired: 2 out]
                n169 = call "Fast_string_Replace.vi"("Replace match with:"="_", "Input String"=w327, "regular expression"="-") -> ("Output String"=w324:string)  [unwired: 2 out]
                n170 = Empty String/Path?(string/path=w324) -> (empty?=w326:bool)
                n171 = case shown="False" w326 {
                  tunnel: [w334 w338] -> w325
                  tunnel: w322 -> [w337 w338]
                  tunnel: w324 -> [w335 _]
                  frame False {
                    n172 = Concatenate Strings(w337, "-" ("string"), w335) -> (w334:string)
                  }
                  frame True {
                  }
                }
              }
            }
          }
          frame True {
          }
        }
        n173 = global write "Preference_global.vi" "Rig Setup"(w283) -> ()
      }
      frame "Update Rig setup menu ring" {
        n174 = local read "Data Folder"() -> (w346:path)
        n175 = Build Path(base path=w346, name or relative path="Preferences") -> (appended path=w345:path)
        n176 = Build Path(base path=w345, name or relative path=w343) -> (appended path=w344:path)
        n177 = List Folder(path=w344) -> (folder names=w342:string[])  [unwired: 1 in, 5 out]
        n178 = Build Array (concatenate)(w342, "--New Rig Setup--") -> (w348:string[])
        n179 = global read "Preference_global.vi" "Rig Setup"() -> (w352:string)
        n180 = Search 1D Array(1D array=w348, element=w352) -> (index of element=w351:i32)  [unwired: 1 out]
        n181 = case shown="-1" w351 {
          selector: w351 -> [w357 _]
          tunnel: [w357 0] -> w354
          tunnel: w348 -> [w358 w361]
          tunnel: w352 -> [_ w360]
          tunnel: [w358 w359] -> w350
          frame 0, Default {
          }
          frame -1 {
            n182 = Build Array (concatenate)(w360, w361) -> (w359:string[])
          }
        }
        n183 = local write "Rig Setup"(w354) -> ()
        n184 = property on="Rig Setup" class="Ring (strict)"("Strings []"=w350) -> ()  [unwired: 2 in, 2 out]
      }
      frame "Update Constants Global" {
        n185 = global read "Constants_global.vi" "Data Folder"() -> (w370:path)
        n186 = Build Path(base path=w370, name or relative path="Preferences") -> (appended path=w373:path)
        n187 = global read "Preference_global.vi" "Rig Setup"() -> (w371:string)
        n188 = Build Path(base path=w373, name or relative path=w372) -> (appended path=w374:path)
        n189 = Build Path(base path=w374, name or relative path=w371) -> (appended path=w367:path)
        n190 = Build Path(base path=w367, name or relative path="ADAM table") -> (appended path=w378:path)
        n191 = Build Path(base path=w367, name or relative path="Serial") -> (appended path=w377:path)
        n192 = Build Path(base path=w367, name or relative path="All_Users") -> (appended path=w366:path)
        n193 = Build Path(base path=w373, name or relative path="Traverse_Setups") -> (appended path=w363:path)
        n194 = Build Path(base path=w366, name or relative path="Collision_detection") -> (appended path=w364:path)
        n195 = global write "Constants_global.vi" "ADAM setups folder"(w378) -> ()
        n196 = global write "Constants_global.vi" "Serial setups folder"(w377) -> ()
        n197 = global write "Constants_global.vi" "Collision_detection"(w364) -> ()
        n198 = global write "Constants_global.vi" "Traverse folder"(w363) -> ()
        n199 = global write "Constants_global.vi" "All_Users"(w366) -> ()
        n200 = Build Array(w363, w378, w377, w366) -> (w376:path[])
        n201 = for {
          tunnel: w376 -> [w387] mode=indexing
          n202 = Build Path(base path=w387, name or relative path="Test") -> (appended path=w385:path)
          n203 = call "Create_directory_path.vi"("Path name"=w385) -> ()  [unwired: 2 in, 2 out]
        }
      }
      frame "Post Processing Machine" {
        n204 = global read "Constants_global.vi" "Data Folder Local"() -> (w395:path)
        n205 = global read "Preference_global.vi" "User_Name"() -> (w390:string)
        n206 = Build Path(base path=w395, name or relative path="Preferences") -> (appended path=w397:path)
        n207 = Build Path(base path=w397, name or relative path=w390) -> (appended path=w391:path)
        n208 = Build Path(base path=w397, name or relative path="Traverse_Setups") -> (appended path=w388:path)
        n209 = Build Path(base path=w391, name or relative path="ADAM table") -> (appended path=w401:path)
        n210 = Build Path(base path=w391, name or relative path="Serial") -> (appended path=w400:path)
        n211 = Build Path(base path=w391, name or relative path="All_Users") -> (appended path=w392:path)
        n212 = global write "Constants_global.vi" "ADAM setups folder"(w401) -> ()
        n213 = global write "Constants_global.vi" "Serial setups folder"(w400) -> ()
        n214 = global write "Constants_global.vi" "Traverse folder"(w388) -> ()
        n215 = global write "Constants_global.vi" "All_Users"(w392) -> ()
        n216 = local write "Post Processing Machine"(TRUE ("Post Processing Machine")) -> ()
        n217 = global write "Preference_global.vi" "Rig Setup"("Post_Processing_Machine" ("Rig Setup")) -> ()
        n218 = Build Array(w388, w401, w400, w392) -> (w399:path[])
        n219 = for {
          tunnel: w399 -> [w410] mode=indexing
          n220 = Build Path(base path=w410, name or relative path="Test") -> (appended path=w408:path)
          n221 = call "Create_directory_path.vi"("Path name"=w408) -> ()  [unwired: 2 in, 2 out]
        }
      }
      frame "Copy Preferences?" {
        n222 = local read "Preferences for computer"() -> (w411:string)
        n223 = call "Setup_Filepath.vi"("Setup File Type"=Setup_Filetype."General", "Filename in"=w411) -> ("Filename Out"=w414:path)  [unwired: 1 out]
        n224 = call <vilib>:"Check if File or Folder Exists.vi"("path"=w414) -> ("file or folder exists?"=w413:bool)  [unwired: 1 in, 9 out]
        n225 = case shown="True" w413 {
          tunnel: w414 -> [w425 _]
          tunnel: [w423 TRUE ("file or folder exists?")] -> w412
          frame False {
            n226 = Strip Path(path=w425) -> (stripped path=w428:path)  [unwired: 1 out]
            n227 = Build Path(base path=w428, name or relative path="Preferences.xls") -> (appended path=w427:path)
            n228 = Move(source path=w427, 10:w425) -> (3:w424:path)  [unwired: 3 in, 2 out]
            n229 = call <vilib>:"Check if File or Folder Exists.vi"("path"=w424) -> ("file or folder exists?"=w423:bool)  [unwired: 1 in, 9 out]
          }
          frame True {
          }
        }
        n230 = case shown="True" w412 {
          tunnel: [w430 TRUE ("Error?")] -> w416
          frame False {
            n231 = global read "Constants_global.vi" "All_Users"() -> (w432:path)
            n232 = Build Path(base path=w432, name or relative path="Current_Username") -> (appended path=w433:path)
            n233 = call "Read_File_Simple.vi"("Filename"=w433) -> ("Error?"=w430:bool)  [unwired: 4 in, 5 out]
          }
          frame True {
          }
        }
        n234 = Select(t="Install Generic Meas Setup file", s=w416, f="Copy from last user") -> (s? t:f=w419:string)
      }
      frame "Copy from last user" {
        n235 = stacked-sequence {
          seq-local: [w442 _ _ _] -> [_ w459 w468 w480]
          seq-local: [_ w455 _ _] -> [_ _ _ w474]
          seq-local: [_ _ w463 _] -> [_ _ _ w473]
          tunnel: [_ _ _ w472] -> w438
          frame #0 {
            n236 = global read "Constants_global.vi" "All_Users"() -> (w453:path)
            n237 = Seconds To Date/Time() -> (date time rec=w449:T12)  [unwired: 2 out]
            n238 = Unbundle By Name(w449) -> ("year"=w450:i32)
            n239 = Build Path(base path=w453, name or relative path="Current_Username") -> (appended path=w451:path)
            n240 = global read "Constants_global.vi" "Data Folder"() -> (w448:path)
            n241 = global read "Preference_global.vi" "Rig Setup"() -> (w445:string)
            n242 = Number To Decimal String(number=w450) -> (decimal integer string=w447:string)  [unwired: 1 out]
            n243 = call "Read_File_Simple.vi"("Filename"=w451) -> ("string"=w444:string)  [unwired: 4 in, 5 out]
            n244 = Build Array(w447, w445, w444, "Preferences" ("name or relative path")) -> (w446:string[])
            n245 = call "Build_Pathname.vi"("PathElements"=w446, "PathnameIn"=w448) -> ("AppendedPath"=w442:path)
          }
          frame #1 {
            n246 = local read "Preferences for computer"() -> (w454:string)
            n247 = Build Path(base path=w459, name or relative path="General") -> (appended path=w461:path)
            n248 = Build Path(base path=w461, name or relative path=w454) -> (appended path=w460:path)
            n249 = call "Setup_Filepath.vi"("Setup File Type"=Setup_Filetype."General", "Filename in"=w454) -> ("Filename Out"=w457:path)  [unwired: 1 out]
            n250 = Copy(10:w457, 11:w460) -> (0:w456:errorcluster)  [unwired: 3 in, 2 out]
            n251 = Unbundle By Name(w456) -> ("status"=w455:bool)
          }
          frame #2 {
            w466 = "Current_Setup.xls"
            n252 = Build Path(base path=w468, name or relative path="Meas Setups") -> (appended path=w470:path)
            n253 = Build Path(base path=w470, name or relative path=w466) -> (appended path=w469:path)
            n254 = call "Setup_Filepath.vi"("Setup File Type"=Setup_Filetype."Measurement Setups", "Filename in"=w466) -> ("Filename Out"=w465:path)  [unwired: 1 out]
            n255 = Copy(10:w465, 11:w469) -> (0:w464:errorcluster)  [unwired: 3 in, 2 out]
            n256 = Unbundle By Name(w464) -> ("status"=w463:bool)
          }
          frame #3 {
            w478 = "Current_Setup.xls"
            n257 = Build Path(base path=w480, name or relative path="Calib Setups") -> (appended path=w482:path)
            n258 = Build Path(base path=w482, name or relative path=w478) -> (appended path=w481:path)
            n259 = call "Setup_Filepath.vi"("Setup File Type"=Setup_Filetype."Calibration Setups", "Filename in"=w478) -> ("Filename Out"=w477:path)  [unwired: 1 out]
            n260 = Copy(10:w477, 11:w481) -> (0:w476:errorcluster)  [unwired: 3 in, 2 out]
            n261 = Unbundle By Name(w476) -> ("status"=w475:bool)
            n262 = Compound Arithmetic op=OR(w475, w474, w473) -> (w472:bool)
          }
        }
        n263 = Select(t="Install Generic Meas Setup file", s=w438, f="Read SW Preferences") -> (s? t:f=w436:string)
      }
      frame "Install Generic Meas Setup file" {
        n264 = global read "Constants_global.vi" "Run VI Folder"() -> (w494:path)
        n265 = Strip Path(path=w494) -> (stripped path=w492:path)  [unwired: 1 out]
        n266 = Build Path(base path=w492, name or relative path="Templates") -> (appended path=w490:path)
        "Templates" <- w490
        n267 = call "Setup_Filepath.vi"("Setup File Type"=Setup_Filetype."Measurement Setups", "Filename in"="Current_Setup.xls" ("name or relative path")) -> ("Filename Out"=w484:path)  [unwired: 1 out]
        n268 = call "Does_file_exist_(simple).vi"("Pathname"=w484) -> ("exists?"=w491:bool)
        n269 = case shown="False" w491 {
          tunnel: w484 -> [w500 _]
          tunnel: w490 -> [w498 _]
          frame False {
            n270 = Build Path(base path=w498, name or relative path="Measurement Setup.xls") -> (appended path=w497:path)
            n271 = Copy(10:w500, 11:w497) -> ()  [unwired: 1 in, 5 out]
          }
          frame True {
          }
        }
        n272 = Build Array (concatenate)(w487, w484) -> (w488:path[])
      }
      frame "Install Preference files" {
        n273 = local read "Preferences for computer"() -> (w501:string)
        n274 = Build Array(w501, w505, "Month_Names.xls" ("name or relative path"), "LDA_Configuration.xls") -> (w509:string[])
        n275 = for {
          tunnel: w509 -> [w513] mode=indexing
          tunnel: [w512] -> w503 mode=indexing
          n276 = call "Setup_Filepath.vi"("Setup File Type"=Setup_Filetype."General", "Filename in"=w513) -> ("Filename Out"=w512:path)  [unwired: 1 out]
          n277 = call "Does_file_exist_(simple).vi"("Pathname"=w512) -> ("exists?"=w515:bool)
          n278 = case shown="True" w515 {
            tunnel: w512 -> [w519 _]
            tunnel: w513 -> [w516 _]
            frame False {
              n279 = local read "Templates"() -> (w517:path)
              n280 = Build Path(base path=w517, name or relative path=w516) -> (appended path=w518:path)
              n281 = Copy(10:w519, 11:w518) -> ()  [unwired: 1 in, 5 out]
            }
            frame True {
            }
          }
        }
        n282 = Build Array (concatenate)(w504, w503) -> (w502:path[])
      }
      frame "Install Adam table files" {
        w524 = "Current_Setup.xls"
        n283 = global read "Constants_global.vi" "ADAM setups folder"() -> (w526:path)
        n284 = Build Path(base path=w526, name or relative path="Setup_Files") -> (appended path=w522:path)
        n285 = Build Path(base path=w522, name or relative path=w524) -> (appended path=w521:path)
        n286 = Build Path(base path=w526, name or relative path=w524) -> (appended path=w527:path)
        n287 = call "Create_directory_path.vi"("Path name"=w521) -> ("Path name Out"=w520:path)  [unwired: 2 in, 1 out]
        n288 = Move(source path=w527, 10:w520) -> ()  [unwired: 1 in, 5 out]
        n289 = Build Array("Hi_Tec_Calibs.xls" ("name or relative path"), "A_Tunnel DB setup.xls" ("Substring"), "EnFlo_Tunnel DB setup.xls", "Aero_Tunnel DB setup.xls" ("name or relative path"), "D_Tunnel DB setup.xls") -> (w534:string[])
        n290 = for {
          tunnel: w534 -> [w538] mode=indexing
          tunnel: w526 -> [w539]
          n291 = Build Path(base path=w539, name or relative path=w538) -> (appended path=w537:path)
          n292 = call "Does_file_exist_(simple).vi"("Pathname"=w537) -> ("exists?"=w540:bool)
          n293 = case shown="False" w540 {
            tunnel: w537 -> [w544 _]
            tunnel: w538 -> [w541 _]
            frame False {
              n294 = local read "Templates"() -> (w542:path)
              n295 = Build Path(base path=w542, name or relative path=w541) -> (appended path=w543:path)
              n296 = Copy(10:w544, 11:w543) -> ()  [unwired: 1 in, 5 out]
            }
            frame True {
            }
          }
        }
      }
      frame "Install Adam setup files" {
        w548 = "Current_Setup.xls"
        n297 = global read "Constants_global.vi" "ADAM setups folder"() -> (w550:path)
        n298 = Build Path(base path=w550, name or relative path="Setup_Files") -> (appended path=w547:path)
        n299 = Build Path(base path=w547, name or relative path=w548) -> (appended path=w545:path)
        n300 = call "Does_file_exist_(simple).vi"("Pathname"=w545) -> ("exists?"=w546:bool)
        n301 = case shown="False" w546 {
          tunnel: w545 -> [w561 _]
          tunnel: w548 -> [w559 _]
          frame False {
            n302 = local read "Templates"() -> (w560:path)
            n303 = Build Path(base path=w560, name or relative path="ADAM_Setup_files") -> (appended path=w558:path)
            n304 = Build Path(base path=w558, name or relative path=w559) -> (appended path=w557:path)
            n305 = Copy(10:w561, 11:w557) -> ()  [unwired: 1 in, 5 out]
          }
          frame True {
          }
        }
        n306 = Build Array (concatenate)(w552, w545) -> (w551:path[])
      }
      frame "Choose ADAM Setup file" {
        w570 = "Selected_Filename.txt" ("Substring")
        n307 = global read "Constants_global.vi" "ADAM setups folder"() -> (w574:path)
        n308 = Build Path(base path=w574, name or relative path="Setup_Files") -> (appended path=w571:path)
        n309 = Build Array(w570) -> (w572:string[])
        n310 = Build Path(base path=w571, name or relative path=w570) -> (appended path=w569:path)
        n311 = call "List_files_in_order_of_age.vi"("Files to Hide"=w572, "Folder"=w571) -> ("file names"=w568:string[])
        n312 = call "Read_File_Simple.vi"("Filename"=w569) -> ("string"=w567:string)  [unwired: 2 in, 7 out]
        n313 = Search 1D Array(1D array=w568, element=w567) -> (index of element=w564:i32)  [unwired: 1 out]
        n314 = property on="ADAM Setup File" class="Ring (strict)"("Strings []"=w568) -> ()  [unwired: 2 in, 2 out]
        n315 = Less Than 0?(x=w564) -> (x < 0?=w565:bool)
        n316 = Select(t=0, s=w565, f=w564) -> (s? t:f=w563:i32)
        n317 = local write "ADAM Setup File"(w563) -> ()
      }
      frame "Preference files continued" {
        n318 = Build Array("Hot_Wire_Bridges.txt", "Hot_Wire_Probes.txt", "Pressure_Transducers.txt") -> (w581:string[])
        n319 = for {
          tunnel: w581 -> [w589] mode=indexing
          tunnel: [w588] -> w579 mode=indexing
          n320 = call "Setup_Filepath.vi"("Setup File Type"=Setup_Filetype."Calibration Setups", "Filename in"=w589) -> ("Filename Out"=w588:path)  [unwired: 1 out]
          n321 = call "Does_file_exist_(simple).vi"("Pathname"=w588) -> ("exists?"=w591:bool)
          n322 = case shown="False" w591 {
            tunnel: w588 -> [w595 _]
            tunnel: w589 -> [w592 _]
            frame False {
              n323 = local read "Templates"() -> (w593:path)
              n324 = Build Path(base path=w593, name or relative path=w592) -> (appended path=w594:path)
              n325 = Copy(10:w595, 11:w594) -> ()  [unwired: 1 in, 5 out]
            }
            frame True {
            }
          }
        }
        n326 = Build Array (concatenate)(w580, w579) -> (w578:path[])
      }
      frame "Variable Names" {
        n327 = Build Array("Traverse to Traverse Collision Detection", "DataTranslation Device No.", "PWA Device Serial No.", "Analogue Device Serial No.", "Server address", "Server port number", "LabVIEW Administrators", "SMTP server IP address", "Server Comms", "Default Source Establishment Time (s)", "Temperature", "Abs Press (mbar)", "Default Traverse Name", "Tunnel Speed Control", "Current Overhead Factor", "EnFlo_Data_Central_Repository", "Auto Calib Error fr Previous", "Auto Calib Error fr First", "EnFlo_Data_Folder_Setup", "Use Triangle and Tree Collision Code", "Log Cameras if available", "Cameras to Log") -> (w618:string[])
        n328 = case shown="\"Load, Edit then Save\"" w612 {
          tunnel: ["Load From Preference file" w624 "Save Preference File"] -> w613
          frame "Load Preferences from file" {
          }
          frame "Load, Edit then Save" {
            n329 = local read "OK"() -> (w627:bool)
            n330 = Select(t="Save Preference File", s=w627, f="Load From Preference file") -> (s? t:f=w624:string)
          }
          frame "Save Preferences to file" {
          }
        }
      }
      frame "Load From Preference file" {
        n331 = local read "Preferences for computer"() -> (w629:string)
        n332 = call "Setup_Filepath.vi"("Setup File Type"=Setup_Filetype."General", "Filename in"=w629) -> ("Filename Out"=w630:path)  [unwired: 1 out]
        n333 = call "Read_File_Simple.vi"("Filename"=w630) -> ("string"=w638:string)  [unwired: 2 in, 7 out]
        n334 = for {
          tunnel: w640 -> [w643] mode=indexing
          tunnel: w638 -> [w642]
          w645 = FALSE  # Show Dialog?
          n335 = call "Get_Characters_from_string.vi"("Show Dialog?"=w645, "Input string"=w642, "Variable name"=w643) -> ("Status"=w644:enum16{"Char in string", "Char not in string"}, "Value"=w641:string)
          n336 = case shown="\"Char in string\"" w644 {
            tunnel: w643 -> [w647 _]
            tunnel: w641 -> [w646 _]
            frame "Char in string" {
              n337 = case shown="\"Abs Press (mbar)\"" w647 {
                selector: w647 -> [w648 _ _ _ _ _ _ _ _ _ _ _ _ _ _ _ _ _ _ _ _ _ _]
                tunnel: w646 -> [_ w650 w651 w654 w655 w658 w659 w660 w662 w664 w667 w670 w673 w676 w678 w679 w682 w686 w687 w689 w691 w694 w696]
                frame "No Match", Default {
                  n338 = call "Was_string_matched.vi"("Match Error"=TRUE, "Variable name"=w648) -> ()  [unwired: 1 in]
                }
                frame "Server address" {
                  n339 = global write "Preference_global.vi" "Server address"(w650) -> ()
                  n340 = local write "Server address"(w650) -> ()
                }
                frame "EnFlo_Data_Folder_Setup" {
                  n341 = local write "EnFlo_Data_Folder_Setup"(w651) -> ()
                  n342 = global write "Preference_global.vi" "EnFlo_Data_Folder_Setup"(w651) -> ()
                }
                frame "DataTranslation Device No." {
                  n343 = Decimal String To Number(string=w654, default (0L)=u32 0 ("default (0 I32)")) -> (number=w652:u32)  [unwired: 1 in, 1 out]
                  n344 = global write "Preference_global.vi" "DataTranslation Device No."(w652) -> ()
                  n345 = local write "DataTranslation Device No."(w652) -> ()
                }
                frame "Default Traverse Name" {
                  n346 = global write "Trav_pos_global.vi" "Default Traverse Setup"(w655) -> ()
                }
                frame "Server port number" {
                  n347 = Decimal String To Number(string=w658) -> (number=w657:i32)  [unwired: 3 out]
                  n348 = To Unsigned Long Integer(number=w657) -> (unsigned 32bit integer=w656:u32)
                  n349 = local write "Server port number"(w656) -> ()
                  n350 = global write "Preference_global.vi" "Server port number"(w656) -> ()
                }
                frame "Analogue Device Serial No." {
                  n351 = local write "Analogue Device Serial No."(w659) -> ()
                }
                frame "PWA Device Serial No." {
                  n352 = local write "PWA Device Serial No."(w660) -> ()
                }
                frame "Default Source Establishment Time (s)" {
                  n353 = Fract/Exp String To Number(string=w662) -> (number=w661:dbl)  [unwired: 4 out]
                  n354 = global write "Preference_global.vi" "Default Source Establishment Time (s)"(w661) -> ()
                  n355 = local write "Default Source Establishment Time (s)"(w661) -> ()
                }
                frame "Tunnel Speed Control" {
                  n356 = Equal?(x="TRUE", y=w664) -> (x = y?=w663:bool)
                  n357 = local write "Tunnel Speed Control"(w663) -> ()
                  n358 = global write "Preference_global.vi" "Tunnel Speed Control"(w663) -> ()
                }
                frame "Traverse to Traverse Collision Detection" {
                  n359 = Equal?(x="TRUE", y=w667) -> (x = y?=w666:bool)
                  n360 = local write "Traverse to Traverse Collision Detection"(w666) -> ()
                  n361 = global write "Preference_global.vi" "Traverse to Traverse Collision Detection"(w666) -> ()
                }
                frame "Log Cameras if available" {
                  n362 = Equal?(x="TRUE", y=w670) -> (x = y?=w669:bool)
                  n363 = global write "Preference_global.vi" "Log Cameras if available"(w669) -> ()
                  n364 = local write "Log Cameras if available"(w669) -> ()
                }
                frame "Use Triangle and Tree Collision Code" {
                  n365 = Equal?(x="TRUE", y=w673) -> (x = y?=w672:bool)
                  n366 = global write "Preference_global.vi" "Use New Collision Code"(w672) -> ()
                  n367 = local write "Use New Collision Code"(w672) -> ()
                }
                frame "LabVIEW Administrators" {
                  n368 = call "Get_array_values_fr_String.vi"("String Value"=w676) -> ("String array"=w675:string[])  [unwired: 1 out]
                  n369 = global write "Preference_global.vi" "LabVIEW Administrators"(w675) -> ()
                  n370 = local write "LabVIEW Administrators"(w675) -> ()
                }
                frame "Cameras to Log" {
                  n371 = call "Get_array_values_fr_String.vi"("String Value"=w678) -> ("String array"=w677:string[])  [unwired: 1 out]
                  n372 = local write "Cameras to Log"(w677) -> ()
                  n373 = global write "CamServer global.vi" "Demanded cameras"(w677) -> ()
                }
                frame "SMTP server IP address" {
                  n374 = local write "SMTP server IP address"(w679) -> ()
                  n375 = global write "Preference_global.vi" "SMTP server IP address"(w679) -> ()
                }
                frame "Server Comms" {
                  n376 = Equal?(x="TRUE", y=w682) -> (x = y?=w681:bool)
                  n377 = case shown="False" w681 {
                    tunnel: [Server_Comms."Do Not Link To Server" ("Server Comms") Server_Comms."Server Link Healthy" ("Server Comms")] -> w680
                    frame False {
                    }
                    frame True {
                    }
                  }
                  n378 = local write "Server Comms"(w680) -> ()
                  n379 = global write "Preference_global.vi" "Server Comms"(w680) -> ()
                }
                frame "Temperature" {
                  n380 = global write "Preference_global.vi" "Temperature"(w686) -> ()
                  n381 = local write "Temperature"(w686) -> ()
                }
                frame "Abs Press (mbar)" {
                  n382 = global write "Preference_global.vi" "Abs Press (mbar)"(w687) -> ()
                  n383 = local write "Abs Press (mbar)"(w687) -> ()
                }
                frame "EnFlo_Data_Central_Repository" {
                  n384 = String To Path(string=w689) -> (path=w688:path)
                  n385 = global write "Constants_global.vi" "EnFlo_Data_Central_Repository"(w688) -> ()
                }
                frame "Current Overhead Factor" {
                  n386 = Fract/Exp String To Number(string=w691) -> (number=w690:dbl)  [unwired: 4 out]
                  n387 = call "Overhead_Factor.vi"("Current Overhead Factor In"=w690, "Mode"=Overhead."Initialise totals to 3hr") -> ()  [unwired: 2 in, 1 out]
                }
                frame "Auto Calib Error fr Previous" {
                  n388 = Fract/Exp String To Number(string=w694) -> (number=w693:dbl)  [unwired: 4 out]
                  n389 = global write "Preference_global.vi" "% Error From Previous Calib"(w693) -> ()
                  n390 = local write "% Error From Previous Calib"(w693) -> ()
                }
                frame "Auto Calib Error fr First" {
                  n391 = Fract/Exp String To Number(string=w696) -> (number=w695:dbl)  [unwired: 4 out]
                  n392 = global write "Preference_global.vi" "% Error From First Calib"(w695) -> ()
                  n393 = local write "% Error From First Calib"(w695) -> ()
                }
              }
            }
            frame "Char not in string" {
            }
          }
        }
        n394 = local read "Post Processing Machine"() -> (w635:bool)
        n395 = Select(t="Check file permission status", s=w635, f="is traverse setup blank?") -> (s? t:f=w633:string)
        n396 = Build Array (concatenate)(w637, w630) -> (w636:path[])
      }
      frame "is traverse setup blank?" {
        n397 = local read "Data Folder"() -> (w703:path)
        n398 = Build Path(base path=w703, name or relative path="Preferences") -> (appended path=w702:path)
        n399 = global read "Trav_pos_global.vi" "Default Traverse Setup"() -> (w697:string)
        n400 = Build Path(base path=w702, name or relative path=w706) -> (appended path=w701:path)
        n401 = List Folder(path=w701) -> (folder names=w699:string[])  [unwired: 1 in, 5 out]
        n402 = Search 1D Array(1D array=w699, element=w697) -> (index of element=w700:i32)  [unwired: 1 out]
        n403 = case shown="0, Default" w700 {
          tunnel: w699 -> [_ w712]
          tunnel: [w710 w711] -> w698
          tunnel: w697 -> [w710 _]
          frame 0, Default {
          }
          frame -1 {
            n404 = Index Array(array=w712, index=0) -> (element=w711:string)
          }
        }
        n405 = global write "Trav_pos_global.vi" "Default Traverse Setup"(w698) -> ()
      }
      frame "Please Enter new  Traverse Setup" {
        n406 = global read "Trav_pos_global.vi" "Default Traverse Setup"() -> (w716:string)
        n407 = String Length(string=w716) -> (length=w721:i32)
        n408 = In Range and Coerce(upper limit=w718, x=w721, lower limit=w719) -> (In Range?=w717:bool)  [unwired: 1 out]
        n409 = case shown="False" w717 {
          tunnel: w716 -> [w732 w740]
          tunnel: ["Please Enter new  Traverse Setup" "Update Traverse setup menu ring"] -> w720
          tunnel: [w725 w740] -> w715
          tunnel: w719 -> [w729 _]
          tunnel: w718 -> [w728 _]
          frame False {
            n410 = Format Into String(format string="Please Enter a Traverse Setup Name\nIt must be between %d and %d Characters" ("Message to user"), w729, w728) -> (resulting string=w727:string)  [unwired: 2 in, 1 out]
            n411 = call "Input_String_Dialog.vi"("Value"=w732, "Message to user"=w727) -> ("Ok Out"=w724:bool, "Output string"=w726:string)
            n412 = case shown="False" w724 {
              tunnel: w726 -> [_ w737]
              tunnel: [w733 w736] -> w725
              frame False {
                n413 = property on="Default Traverse Name" class="Ring (strict)"() -> ("Strings []"=w734:string[])  [unwired: 2 in, 2 out]
                n414 = Index Array(array=w734, index=0) -> (element=w733:string)
              }
              frame True {
                n415 = call "Fast_string_Replace.vi"("Replace match with:"="_", "Input String"=w737, "regular expression"=" ") -> ("Output String"=w736:string)  [unwired: 2 out]
              }
            }
          }
          frame True {
          }
        }
        n416 = global write "Trav_pos_global.vi" "Default Traverse Setup"(w715) -> ()
      }
      frame "Update Traverse setup menu ring" {
        n417 = local read "Data Folder"() -> (w751:path)
        n418 = Build Path(base path=w751, name or relative path="Preferences") -> (appended path=w750:path)
        n419 = Build Path(base path=w750, name or relative path=w743) -> (appended path=w749:path)
        n420 = global read "Trav_pos_global.vi" "Default Traverse Setup"() -> (w745:string)
        n421 = List Folder(path=w749) -> (folder names=w747:string[])  [unwired: 1 in, 5 out]
        n422 = Build Array (concatenate)(w747, "--New Traverse Setup--") -> (w746:string[])
        n423 = Search 1D Array(1D array=w746, element=w745) -> (index of element=w753:i32)  [unwired: 1 out]
        n424 = case shown="-1" w753 {
          selector: w753 -> [w758 _]
          tunnel: [w758 0] -> w755
          tunnel: w746 -> [w759 w762]
          tunnel: w745 -> [_ w761]
          tunnel: [w759 w760] -> w744
          frame 0, Default {
          }
          frame -1 {
            n425 = Build Array (concatenate)(w761, w762) -> (w760:string[])
          }
        }
        n426 = local write "Default Traverse Name"(w755) -> ()
        n427 = property on="Default Traverse Name" class="Ring (strict)"("Strings []"=w744) -> ()  [unwired: 2 in, 2 out]
      }
      frame "Create Traverse setup" {
        n428 = local read "Templates"() -> (w765:path)
        n429 = Build Path(base path=w765, name or relative path="All_Traverses") -> (appended path=w771:path)
        n430 = stacked-sequence {
          seq-local: [w776 _] -> [_ w804]
          seq-local: [w775 _] -> [_ _]
          tunnel: w771 -> [w778 _]
          tunnel: [w781 _] -> w768
          tunnel: [w780 _] -> w767
          tunnel: w765 -> [_ w803]
          tunnel: [_ w801] -> w764
          frame #0 {
            w784 = "Default_Space_file.xls" ("name or relative path")
            w779 = "Traverse_Setup.xls" ("name or relative path")
            n431 = global read "Trav_pos_global.vi" "Default Traverse Setup"() -> (w775:string)
            n432 = global read "Constants_global.vi" "Traverse folder"() -> (w788:path)
            n433 = Build Path(base path=w778, name or relative path=w784) -> (appended path=w782:path)
            n434 = Build Path(base path=w778, name or relative path=w779) -> (appended path=w777:path)
            n435 = Build Path(base path=w788, name or relative path=w775) -> (appended path=w776:path)
            n436 = Build Path(base path=w776, name or relative path="Trav_Space_Files") -> (appended path=w785:path)
            n437 = Build Path(base path=w785, name or relative path=w784) -> (appended path=w781:path)
            n438 = call "Does_file_exist_(simple).vi"("Pathname"=w781) -> ("exists?"=w783:bool)
            n439 = case shown="False" w783 {
              tunnel: w782 -> [w791 _]
              tunnel: w781 -> [w790 _]
              frame False {
                n440 = call "Create_directory_path.vi"("Path name"=w790) -> ("Path name Out"=w789:path)  [unwired: 2 in, 1 out]
                n441 = Copy(10:w789, 11:w791) -> ()  [unwired: 1 in, 5 out]
              }
              frame True {
              }
            }
            n442 = Build Path(base path=w776, name or relative path=w779) -> (appended path=w780:path)
            n443 = call "Does_file_exist_(simple).vi"("Pathname"=w780) -> ("exists?"=w787:bool)
            n444 = case shown="False" w787 {
              tunnel: w777 -> [w800 _]
              tunnel: w780 -> [w796 _]
              tunnel: w775 -> [w799 _]
              frame False {
                w792 = TRUE  # append to file? (new file:F)
                n445 = call "Create_directory_path.vi"("Path name"=w796) -> ("Path name Out"=w795:path)  [unwired: 2 in, 1 out]
                n446 = call "Read_File_Simple.vi"("Filename"=w800) -> ("string"=w798:string)  [unwired: 2 in, 7 out]
                n447 = call "Fast_string_Replace.vi"("Replace match with:"=w799, "Input String"=w798, "regular expression"="A_Tunnel") -> ("Output String"=w794:string)  [unwired: 2 out]
                n448 = call "Write_Characters_To_File.vi"("file path (dialog if empty)"=w795, "advisory dialog? (display:T)"=TRUE, "character string"=w794, "append to file? (new file:F)"=w792) -> ()  [unwired: 1 in, 4 out]
              }
              frame True {
              }
            }
          }
          frame #1 {
            w802 = "Traverse_Preferences.txt" ("name or relative path")
            n449 = Build Path(base path=w804, name or relative path=w802) -> (appended path=w801:path)
            n450 = Build Path(base path=w803, name or relative path=w802) -> (appended path=w805:path)
            n451 = call "Does_file_exist_(simple).vi"("Pathname"=w801) -> ("exists?"=w806:bool)
            n452 = case shown="False" w806 {
              tunnel: w805 -> [w809 _]
              tunnel: w801 -> [w808 _]
              frame False {
                n453 = call "Create_directory_path.vi"("Path name"=w808) -> ("Path name Out"=w807:path)  [unwired: 2 in, 1 out]
                n454 = Copy(10:w807, 11:w809) -> ()  [unwired: 1 in, 5 out]
              }
              frame True {
              }
            }
          }
        }
        n455 = Build Array (concatenate)(w770, w767, w764, w768) -> (w769:path[])
      }
      frame "Check file permission status" {
        n456 = local read "Post Processing Machine"() -> (w810:bool)
        n457 = for {
          tunnel: w815 -> [w829] mode=indexing
          shift-right: [w826] -> w812
          shift-left: "" -> [w827]
          n458 = call "Can_File_be_Editted.vi"("Filename"=w829) -> ("File Permissions OK?"=w830:bool, "Comment String"=w828:string)  [unwired: 2 out]
          n459 = case shown="False" w830 {
            tunnel: w829 -> [w835 _]
            tunnel: w828 -> [w834 _]
            tunnel: w827 -> [w833 w836]
            tunnel: [w832 w836] -> w826
            frame False {
              n460 = Format Into String(format string="\"%s\" %s\n", initial string=w833, w835, w834) -> (resulting string=w832:string)  [unwired: 1 in, 1 out]
            }
            frame True {
            }
          }
        }
        n461 = case shown="\"Load, Edit then Save\"" w816 {
          tunnel: [w838 w842] -> w817
          tunnel: w810 -> [w837 w841]
          frame "Save Preferences to file", Default {
            n462 = Select(t="Save Preference File", s=w837, f="Output Dev Number") -> (s? t:f=w838:string)
          }
          frame "Load, Edit then Save" {
            n463 = Select(t="Data Folder Changed?", s=w841, f="What next1") -> (s? t:f=w842:string)
          }
        }
        n464 = Empty String/Path?(string/path=w812) -> (empty?=w813:bool)
        n465 = case shown="True" w813 {
          tunnel: w812 -> [w825 _]
          frame False {
            n466 = Concatenate Strings("The following file permissions need to be sorted out before the software will run correctly.\n\n" ("string"), w825) -> (w823:string)
            n467 = Two Button Dialog(message=w823, 1:"Continue" ("F button name (\"Cancel\")"), 2:"Abort" ("F button name (\"Cancel\")")) -> (T button?=w820:bool)
            n468 = Stop(stop? (T)=w820) -> ()
          }
          frame True {
          }
        }
      }
      frame "What next1" {
        n469 = property on="Rig Setup" class="Ring (strict)"() -> ("Strings []"=w847:string[])  [unwired: 2 in, 2 out]
        n470 = Array Size(array=w847) -> (size(s)=w851:i32)
        n471 = Decrement(x=w851) -> (x-1=w850:i32)
        n472 = Equal?(x=w850, y="Rig Setup") -> (x = y?=w849:bool)
        n473 = case shown="False" w849 {
          tunnel: [w855 "Please Enter New Rig Name" ("t")] -> w848
          tunnel: w847 -> [w858 _]
          tunnel: "Rig Setup" -> [w857 _]
          frame False {
            n474 = global read "Preference_global.vi" "Rig Setup"() -> (w859:string)
            n475 = Index Array(array=w858, index=w857) -> (element=w854:string)
            n476 = Not Equal?(x=w854, y=w859) -> (x != y?=w856:bool)
            n477 = case shown="False" w856 {
              tunnel: ["What next2" ("f") "Update Rig setup menu ring" ("t")] -> w855
              tunnel: w854 -> [_ w861]
              frame False {
              }
              frame True {
                n478 = global write "Preference_global.vi" "Rig Setup"(w861) -> ()
              }
            }
          }
          frame True {
            n479 = global write "Preference_global.vi" "Rig Setup"("") -> ()
          }
        }
      }
      frame "What next2" {
        n480 = property on="Default Traverse Name" class="Ring (strict)"() -> ("Strings []"=w867:string[])  [unwired: 2 in, 2 out]
        n481 = Array Size(array=w867) -> (size(s)=w871:i32)
        n482 = Decrement(x=w871) -> (x-1=w870:i32)
        n483 = Equal?(x=w870, y="Default Traverse Name") -> (x = y?=w869:bool)
        n484 = case shown="False" w869 {
          tunnel: [w875 "Please Enter new  Traverse Setup" ("t")] -> w868
          tunnel: w867 -> [w879 _]
          tunnel: "Default Traverse Name" -> [w878 _]
          frame False {
            n485 = global read "Trav_pos_global.vi" "Default Traverse Setup"() -> (w877:string)
            n486 = Index Array(array=w879, index=w878) -> (element=w874:string)
            n487 = Not Equal?(x=w874, y=w877) -> (x != y?=w876:bool)
            n488 = case shown="True" w876 {
              tunnel: ["Data Folder Changed?" ("f") "Update Traverse setup menu ring" ("t")] -> w875
              tunnel: w874 -> [_ w881]
              frame False {
              }
              frame True {
                n489 = global write "Trav_pos_global.vi" "Default Traverse Setup"(w881) -> ()
              }
            }
          }
          frame True {
            n490 = global write "Trav_pos_global.vi" "Default Traverse Setup"("") -> ()
          }
        }
      }
      frame "Data Folder Changed?" {
        w887 = "Please Select your data folder"
        n491 = while {
          shift-right: [w903] -> _
          shift-left: _ -> [w902]
          tunnel: [w901] -> w889
          stop <- TRUE stop-if-true
          n492 = local read "Post Processing Machine"() -> (w903:bool)
          n493 = Not Equal?(x=w903, y=w902) -> (x != y?=w901:bool)
        }
        n494 = global read "Constants_global.vi" "Data Folder"() -> (w893:path)
        n495 = local read "Data Folder"() -> (w894:path)
        n496 = Not Equal?(x=w893, y=w894) -> (x != y?=w885:bool)
        n497 = Select(t=w887, s=w885, f="Has OK has been pressed?") -> (s? t:f=w886:string)
        n498 = case shown="True" w889 {
          tunnel: [w897 w899] -> w888
          tunnel: w887 -> [_ w899]
          tunnel: w886 -> [w897 _]
          frame False {
          }
          frame True {
            n499 = global write "Preference_global.vi" "Rig Setup"("") -> ()
          }
        }
        n500 = property on="OK" class="Bool (strict)"("Visible"=TRUE) -> ()  [unwired: 2 in, 2 out]
      }
      frame "Has OK has been pressed?" {
        n501 = flat-sequence {
          tunnel: ["OK"] -> w905
          frame #0 {
            n502 = Wait (ms)(milliseconds to wait=u32 100) -> ()  [unwired: 1 out]
          }
          frame #1 {
          }
        }
        n503 = local read "Post Processing Machine"() -> (w906:bool)
        n504 = case shown="True" w905 {
          tunnel: w906 -> [w911 w917]
          tunnel: [w910 w914] -> w904
          frame False {
            n505 = Select(t="Data Folder Changed?", s=w911, f="What next1") -> (s? t:f=w910:string)
          }
          frame True {
            n506 = Select(t="Save Preference File", s=w917, f="Output Dev Number") -> (s? t:f=w914:string)
          }
        }
      }
      frame "Output Dev Number" {
        n507 = for {
          tunnel: string[] ["Raw_Calibrations", "Raw_Measurements", "Results", "Calibrations", "Commands", "Pictures", "Videos"] -> [w933] mode=indexing
          tunnel: string[] ["Raw_Cal", "Raw_Meas", "Res", "Cal", "Cmd", "Pic", "Video"] -> [w931] mode=indexing
          n508 = call "Data_folder_Path.vi"("Data Type"=w933, "Short_Name"=w931) -> ("Data Folder"=w932:path)  [unwired: 4 in]
          n509 = Build Path(base path=w932, name or relative path="Test" ("Substring")) -> (appended path=w935:path)
          n510 = call "Create_directory_path.vi"("Path name"=w935) -> ()  [unwired: 2 in, 2 out]
        }
        n511 = local read "Analogue Device Serial No."() -> (w925:string)
        n512 = call "Data_folder_Path.vi"("Data Type"="Results_Post_Processed" ("element"), "Short_Name"="PP" ("ProjectNumberIn")) -> ("Data Folder"=w922:path)  [unwired: 4 in]
        n513 = local read "PWA Device Serial No."() -> (w926:string)
        n514 = call "Create_directory_path.vi"("Path name"=w922) -> ()  [unwired: 2 in, 2 out]
        n515 = global write "PWAtasksGLOBAL.vi" "PWA Dev Name"(w926) -> ()
        n516 = global write "PWAtasksGLOBAL.vi" "Analogue Dev Name"(w925) -> ()
      }
      frame "Save Preference File" {
        n517 = call "Date_and_Time_to_string.vi"() -> ("Date and time (spreadsheet)"=w947:string)
        n518 = for {
          tunnel: w946 -> [w957] mode=indexing
          shift-right: [w953] -> w945
          shift-left: w947 -> [w955]
          n519 = case shown="\"Cameras to Log\"" w957 {
            selector: w957 -> [w958 _ _ _ _ _ _ _ _ _ _ _ _ _ _ _ _ _ _ _ _ _ _]
            tunnel: ["No Match" "Server address" "EnFlo_Data_Folder_Setup" w964 w966 w968 w972 w976 w980 w984 w988 "SMTP server IP address" "PWA Device Serial No." "Analogue Device Serial No." w996 w997 w999 "Temperature" "Abs Press (mbar)" w1004 w1009 w1012 w1015] -> w956
            frame "No Match", Default {
              n520 = call "Was_string_matched.vi"("Match Error"=TRUE, "Variable name"=w958) -> ()  [unwired: 1 in]
            }
            frame "Server address" {
              n521 = global write "Preference_global.vi" "Server address"("Server address") -> ()
            }
            frame "EnFlo_Data_Folder_Setup" {
              n522 = global write "Preference_global.vi" "EnFlo_Data_Folder_Setup"("EnFlo_Data_Folder_Setup") -> ()
            }
            frame "Server port number" {
              n523 = global write "Preference_global.vi" "Server port number"("Server port number") -> ()
              n524 = Number To Decimal String(number="Server port number") -> (decimal integer string=w964:string)  [unwired: 1 out]
            }
            frame "Default Source Establishment Time (s)" {
              n525 = global write "Preference_global.vi" "Default Source Establishment Time (s)"("Default Source Establishment Time (s)") -> ()
              n526 = Number To Decimal String(number="Default Source Establishment Time (s)") -> (decimal integer string=w966:string)  [unwired: 1 out]
            }
            frame "Tunnel Speed Control" {
              n527 = global write "Preference_global.vi" "Tunnel Speed Control"("Tunnel Speed Control") -> ()
              n528 = Select(t="TRUE", s="Tunnel Speed Control", f="FALSE") -> (s? t:f=w968:string)
            }
            frame "Traverse to Traverse Collision Detection" {
              n529 = global write "Preference_global.vi" "Traverse to Traverse Collision Detection"("Traverse to Traverse Collision Detection") -> ()
              n530 = Select(t="TRUE", s="Traverse to Traverse Collision Detection", f="FALSE") -> (s? t:f=w972:string)
            }
            frame "Log Cameras if available" {
              n531 = global write "Preference_global.vi" "Log Cameras if available"("Log Cameras if available") -> ()
              n532 = Select(t="TRUE", s="Log Cameras if available", f="FALSE") -> (s? t:f=w976:string)
            }
            frame "Use Triangle and Tree Collision Code" {
              n533 = global write "Preference_global.vi" "Use New Collision Code"("Use New Collision Code") -> ()
              n534 = Select(t="TRUE", s="Use New Collision Code", f="FALSE") -> (s? t:f=w980:string)
            }
            frame "LabVIEW Administrators" {
              n535 = global write "Preference_global.vi" "LabVIEW Administrators"("LabVIEW Administrators") -> ()
              n536 = call "Put_Array_into_String.vi"("String array"="LabVIEW Administrators") -> ("String Value"=w984:string)
            }
            frame "Cameras to Log" {
              n537 = call "Analyse_string_array.vi"("String array"="Cameras to Log") -> ("Unique strings"=w986:string[])  [unwired: 1 in, 1 out]
              n538 = for {
                tunnel: w986 -> [w990] mode=indexing
                tunnel: [w990] -> w985 mode=indexing if=w989
                n539 = Not Equal?(x=w990, y="None") -> (x != y?=w989:bool)
              }
              n540 = global write "CamServer global.vi" "Demanded cameras"(w985) -> ()
              n541 = call "Put_Array_into_String.vi"("String array"=w985) -> ("String Value"=w988:string)
            }
            frame "SMTP server IP address" {
              n542 = global write "Preference_global.vi" "SMTP server IP address"("SMTP server IP address") -> ()
            }
            frame "PWA Device Serial No." {
            }
            frame "Analogue Device Serial No." {
            }
            frame "DataTranslation Device No." {
              n543 = global write "Preference_global.vi" "DataTranslation Device No."("DataTranslation Device No.") -> ()
              n544 = Number To Decimal String(number="DataTranslation Device No.") -> (decimal integer string=w996:string)  [unwired: 1 in]
            }
            frame "Default Traverse Name" {
              n545 = global read "Trav_pos_global.vi" "Default Traverse Setup"() -> (w997:string)
            }
            frame "Server Comms" {
              n546 = case shown="\"Server Link Healthy\"" "Server Comms" {
                tunnel: ["TRUE" "FALSE"] -> w999
                frame "Server Link Healthy" {
                }
                frame "Do Not Link To Server" {
                }
              }
              n547 = global write "Preference_global.vi" "Server Comms"("Server Comms") -> ()
            }
            frame "Temperature" {
              n548 = global write "Preference_global.vi" "Temperature"("Temperature") -> ()
            }
            frame "Abs Press (mbar)" {
              n549 = global write "Preference_global.vi" "Abs Press (mbar)"("Abs Press (mbar)") -> ()
            }
            frame "Current Overhead Factor" {
              n550 = call "Overhead_Factor.vi"("Mode"=Overhead."Read Current Overhead") -> ("Current Overhead Factor"=w1006:dbl)  [unwired: 3 in]
              n551 = Number To Fractional String(number=w1006, precision (6)=i16 4) -> (F-format string=w1004:string)  [unwired: 2 out]
            }
            frame "Auto Calib Error fr Previous" {
              n552 = global write "Preference_global.vi" "% Error From Previous Calib"("% Error From Previous Calib") -> ()
              n553 = Number To Fractional String(number="% Error From Previous Calib", precision (6)=i16 2) -> (F-format string=w1009:string)  [unwired: 2 out]
            }
            frame "Auto Calib Error fr First" {
              n554 = global write "Preference_global.vi" "% Error From First Calib"("% Error From First Calib") -> ()
              n555 = Number To Fractional String(number="% Error From First Calib", precision (6)=i16 2) -> (F-format string=w1012:string)  [unwired: 2 out]
            }
            frame "EnFlo_Data_Central_Repository" {
              n556 = global read "Constants_global.vi" "EnFlo_Data_Central_Repository"() -> (w1014:path)
              n557 = Path To String(path=w1014) -> (string=w1015:string)
            }
          }
          n558 = call "Characters_to_string.vi"("Characters to write"=w956, "Label for characters"=w957) -> ("Output string"=w954:string)
          n559 = Concatenate Strings(w955, w954) -> (w953:string)
        }
        n560 = case shown="\"Load, Edit then Save\"" w941 {
          tunnel: [TRUE TRUE TRUE] -> w940
          frame "Load, Edit then Save" {
            n561 = Current VI's Path() -> (path=w949:path)
            n562 = call "Open_Close_Front_Panel.ph.vi"("Front Panel Window:Open"=FALSE, "VI path"=w949) -> ()  [unwired: 2 out]
          }
          frame "Load Preferences from file" {
          }
          frame "Save Preferences to file" {
          }
        }
        n563 = local read "Preferences for computer"() -> (w936:string)
        n564 = call "Setup_Filepath.vi"("Setup File Type"=Setup_Filetype."General", "Filename in"=w936) -> ("Filename Out"=w937:path)  [unwired: 1 out]
        n565 = call "Write_Characters_To_File.vi"("file path (dialog if empty)"=w937, "advisory dialog? (display:T)"=FALSE, "character string"=w945, "append to file? (new file:F)"=FALSE) -> ()  [unwired: 1 in, 4 out]
      }
      frame "Save SW Preferences" {
        w1035 = FALSE  # append to file? (new file:F)
        w1036 = FALSE  # advisory dialog? (display:T)
        n566 = local read "Post Processing Machine"() -> (w1025:bool)
        n567 = global read "Preference_global.vi" "User_Name"() -> (w1018:string)
        n568 = Path To String(path="Data Folder") -> (string=w1027:string)
        n569 = call "Characters_to_string.vi"("Characters to write"=w1027, "Label for characters"=w1029) -> ("Output string"=w1037:string)
        n570 = Select(t="True", s=w1025, f="False") -> (s? t:f=w1022:string)
        n571 = call "Characters_to_string.vi"("Characters to write"=w1018, "Label for characters"=w1019) -> ("Output string"=w1017:string)
        n572 = call "Characters_to_string.vi"("Characters to write"=w1022, "Label for characters"=w1020) -> ("Output string"=w1021:string)
        n573 = call "Date_and_Time_to_string.vi"() -> ("Date and time (spreadsheet)"=w1032:string)
        n574 = Concatenate Strings(w1032, w1037, w1021, w1017) -> (w1033:string)
        n575 = local read "EnFlo SW Preferences"() -> (w1034:path)
        n576 = call "Write_Characters_To_File.vi"("file path (dialog if empty)"=w1034, "advisory dialog? (display:T)"=w1036, "character string"=w1033, "append to file? (new file:F)"=w1035) -> ()  [unwired: 1 in, 4 out]
        n577 = global read "Preference_global.vi" "Server Comms"() -> (w1031:T4)
        n578 = case shown="\"Server Link Healthy\"" w1031 {
          tunnel: ["Update Served VI file" "Update Local Adam Table"] -> w1030
          frame "Server Link Healthy" {
          }
          frame "Do Not Link To Server" {
          }
        }
        n579 = case shown="True" "Reset Email Counter" {
          tunnel: "Reset Email Counter" -> [_ w1040]
          frame False {
          }
          frame True {
            n580 = global write "Preference_global.vi" "Unblock Email"(w1040) -> ()
          }
        }
      }
      frame "Update Local Adam Table" {
        n581 = stacked-sequence {
          seq-local: [w1052 _] -> [_ w1066]
          tunnel: ["Update Served VI file" _] -> w1044
          frame #0 {
            w1052 = T13 {"Ch Name"="", "Type"="", "Function"=enum."Analogue Input", "Ch State"=enum."On", "Calibration type"=enum."Raw", "A"=0.0, "B"=0.0, "C"=0.0, "D"=0.0, "Comments"="", "Address"={"Main"=0, "Ch."=0, "Sub"=0, "Port Name"=""}, "String"="", "Duty"=0} ("Ch Discription")
            n582 = global read "Preference_global.vi" "Abs Press (mbar)"() -> (w1049:string)
            n583 = global read "Preference_global.vi" "Temperature"() -> (w1050:string)
            n584 = Bundle By Name(cluster=w1052, "Type"=T10 "", "Calibration type"=Calib_type_ADAM."Raw", "A"=1.0) -> (w1053:T13)
            n585 = Build Array(w1050, w1049) -> (w1048:string[])
            n586 = for {
              tunnel: [w1059] -> w1051 mode=indexing
              tunnel: w1053 -> [w1058]
              tunnel: w1048 -> [w1057] mode=indexing
              n587 = Bundle By Name(cluster=w1058, "Ch Name"=w1057) -> (w1059:T13)
            }
            n588 = call "Update_Ch_Discription_client.vi"("Channels to update In"=w1051) -> ()  [unwired: 1 out]
          }
          frame #1 {
            n589 = global read "Preference_global.vi" "Rig Setup"() -> (w1061:string)
            n590 = call "Get_Current_Scan_client.vi"() -> ("Ch Description Array"=w1067:T13[])  [unwired: 1 in, 3 out]
            n591 = Match Pattern(string=w1061, regular expression="-") -> (before substring=w1060:string)  [unwired: 4 out]
            n592 = Format Into String(format string="%s Metadata:" ("Format String"), w1060) -> (resulting string=w1069:string)  [unwired: 2 in, 1 out]
            n593 = Initialize Array(w1066, 0 ("dimension size")) -> (w1064:T13[])
            n594 = for {
              shift-right: [w1080] -> w1063
              shift-left: w1064 -> [w1081]
              tunnel: w1067 -> [w1072] mode=indexing
              tunnel: w1069 -> [w1079]
              tunnel: "Metadata:" ("Format String") -> [w1078]
              n595 = Unbundle By Name(w1072) -> ("Ch Name"=w1071:string)
              n596 = Match Pattern(string=w1071, regular expression=w1079) -> (offset past match=w1076:i32)  [unwired: 4 out]
              n597 = Match Pattern(string=w1071, regular expression=w1078) -> (offset past match=w1077:i32)  [unwired: 4 out]
              n598 = Greater Or Equal To 0?(x=w1077) -> (x >= 0?=w1074:bool)
              n599 = Less Than 0?(x=w1076) -> (x < 0?=w1075:bool)
              n600 = And(x=w1075, y=w1074) -> (x .and. y?=w1073:bool)
              n601 = case shown="True" w1073 {
                tunnel: w1081 -> [w1082 w1087]
                tunnel: [w1082 w1086] -> w1080
                tunnel: w1072 -> [_ w1085]
                frame False {
                }
                frame True {
                  n602 = Bundle By Name(cluster=w1085, "Ch State"=Channel_State."Off") -> (w1083:T13)
                  n603 = Build Array (concatenate)(w1087, w1083) -> (w1086:T13[])
                }
              }
            }
            n604 = call "Update_Ch_Discription_client.vi"("Channels to update In"=w1063) -> ()  [unwired: 1 out]
          }
        }
      }
      frame "Update Served VI file" {
        n605 = call "Setup_Filepath.vi"("Setup File Type"=Setup_Filetype."General", "Filename in"=w1089) -> ("Filename Out"=w1088:path)  [unwired: 1 out]
        n606 = Build Array("Served:VI:Name", "Served:VI:Path", "Server:IP Number:& Port No") -> (w1094:string[])
        n607 = stacked-sequence {
          seq-local: [w1099 _ _ _] -> [_ _ w1109 _]
          seq-local: [_ w1106 _ _] -> [_ _ w1110 _]
          seq-local: [_ _ w1111 _] -> [_ _ _ w1135]
          tunnel: w1094 -> [w1101 w1107 _ w1136]
          tunnel: w1088 -> [w1100 _ _ w1137]
          tunnel: w1089 -> [_ w1103 _ _]
          frame #0 {
            n608 = call "Read_Ch_data_file.vi"("Present Channels"=w1101, "Output"=enum16{"All Ch data", "The last few rows"}."All Ch data", "Filename"=w1100) -> ("Channel Values"=w1099:string[][])  [unwired: 2 in, 4 out]
          }
          frame #1 {
            n609 = local read "Templates"() -> (w1105:path)
            n610 = Build Path(base path=w1105, name or relative path=w1103) -> (appended path=w1104:path)
            n611 = call "Read_Ch_data_file.vi"("Present Channels"=w1107, "Output"=enum16{"All Ch data", "The last few rows"}."All Ch data", "Filename"=w1104) -> ("Channel Values"=w1106:string[][])  [unwired: 2 in, 4 out]
          }
          frame #2 {
            n612 = Index Array(array=w1109, index (col)=0 ("Index")) -> (element=w1114:string[])  [unwired: 1 in]
            n613 = To Upper Case(1:w1110) -> (0:w1112:string[][])
            n614 = To Upper Case(1:w1114) -> (0:w1113:string[])
            n615 = for {
              tunnel: w1113 -> [w1117]
              tunnel: w1110 -> [w1122] mode=indexing
              tunnel: w1112 -> [w1116] mode=indexing
              tunnel: [w1119] -> w1111 mode=indexing
              tunnel: w1109 -> [w1118]
              n616 = Index Array(array=w1116, index=0 ("Index")) -> (element=w1120:string)
              n617 = Search 1D Array(1D array=w1117, element=w1120) -> (index of element=w1121:i32)  [unwired: 1 out]
              n618 = case shown="0, Default" w1121 {
                tunnel: w1122 -> [w1131 w1132]
                tunnel: w1121 -> [w1128 _]
                tunnel: [w1124 w1132] -> w1119
                tunnel: w1118 -> [w1129 _]
                frame 0, Default {
                  n619 = Index Array(array=w1129, index (row)=w1128, index (col)=2 ("Index")) -> (element=w1126:string)
                  n620 = Array Subset(array=w1131, length=2) -> (w1125:string[])  [unwired: 1 in]
                  n621 = Build Array (concatenate)(w1125, w1126) -> (w1124:string[])
                }
                frame -1 {
                }
              }
            }
          }
          frame #3 {
            w1133 = FALSE  # Append last row only
            w1134 = FALSE  # exists?
            n622 = call "Write_Ch_data_file.vi"("Append last row only"=w1133, "exists?"=w1134, "Channel Values"=w1135, "Channel names"=w1136, "Filename"=w1137) -> ()  [unwired: 3 in, 4 out]
          }
        }
      }
      frame "Initialise Globals" {
        w1142 = TRUE  # OK
        w1146 = FALSE  # append to file? (new file:F)
        w1145 = FALSE  # advisory dialog? (display:T)
        n623 = global read "Constants_global.vi" "ADAM setups folder"() -> (w1152:path)
        n624 = property on="ADAM Setup File" class="Ring (strict)"() -> ("Strings []"=w1147:string[])  [unwired: 2 in, 2 out]
        n625 = Build Path(base path=w1152, name or relative path="Setup_Files") -> (appended path=w1150:path)
        n626 = Build Path(base path=w1150, name or relative path="Selected_Filename.txt" ("Substring")) -> (appended path=w1143:path)
        n627 = Index Array(array=w1147, index="ADAM Setup File") -> (element=w1144:string)
        n628 = global read "Constants_global.vi" "All_Users"() -> (w1141:path)
        n629 = Build Path(base path=w1141, name or relative path="Current_Username") -> (appended path=w1139:path)
        n630 = global read "Preference_global.vi" "User_Name"() -> (w1138:string)
        n631 = call "Write_Characters_To_File.vi"("file path (dialog if empty)"=w1143, "advisory dialog? (display:T)"=w1145, "character string"=w1144, "append to file? (new file:F)"=w1146) -> ()  [unwired: 1 in, 4 out]
        n632 = call "Write_File_Simple.vi"("character string"=w1138, "file path"=w1139) -> ()  [unwired: 1 in, 2 out]
        n633 = call "Get_users_email_addresses.vi"("OK"=w1142) -> ()  [unwired: 5 out]
      }
    }
  }
